vi "ASD PowerPoint Main.vi"() -> ()   [LabVIEW 2021]
uses:
  Controls/Functions Tab.ctl
  Controls/Channel Configuration List.ctl
  Controls/Channel Configuration Cluster.ctl
  Controls/Channel Configuration Cluster High Current.ctl
  Controls/Gain Array.ctl
  Controls/WT1800 Measurements.ctl
  Controls/WT1800 Readings.ctl
  Controls/Gain Averages.ctl
  Controls/Consumer Control.ctl
  Controls/Error Module Command.ctl
  Controls/DSA Readings.ctl
  Controls/Datalog Bundle Control.ctl
  Controls/WT1800 Functions.ctl
  Controls/DSA Functions.ctl
  Controls/DSA Measurements.ctl
panel:
  in  "User Gains":T1 {"Gain 6" format="%.2f"; "Gain 5" format="%.2f"; "Gain 4" format="%.2f"; "Gain 3" format="%.2f"; "Gain 2" min=-10.0 max=50.0 step=0.01 format="%.2f"; "Gain 1" min=-10.0 max=50.0 step=0.01 format="%.2f"}
  in  "Stop":bool
  in  "Home":bool
  in  "Abort":bool
  in  "Tab Control":T2
  in  "Power Test M":bool
  in  "Wave File 4":path
  in  "Wave File 3":path
  in  "Supply Set":bool
  in  "Temp Criteria":dbl caption="Temp Convergence Criteria [deg C]" min=0.0 max=10.0 step=0.01 format="%.2f"
  in  "Check EQ":bool
  in  "Load Settings":bool
  in  "Wave File 1":path
  in  "Voltage Steps":dbl[](array[numeric])=[0.0, 0.25, 0.5, 1.0, 1.95, 3.0, 3.9, 5.5] caption="Voltage Steps [Vrms]" min=0.0 max=500.0 step=0.01 format="%.2f"
  in  "User Notes":string
  in  "Supply Amps":dbl=50.0 caption="Max Supply Amps [Idc]" min=5.0 max=50.0 format="%.2f"
  in  "Supply Volts":dbl=14.4 caption="Supply Volts [Vdc]" min=10.0 max=15.0 format="%.2f"
  in  "Save Settings":bool
  in  "Configure Channels":bool
  in  "Exit":bool
  in  "Settling Delay":dbl=10.0 min=0.0 max=86400.0 format="%<%H:%M:%S>t"
  in  "Power Test":bool
  in  "Wave File 2":path
  in  "Data File":path caption="Data File Path"
  in  "Crest Factor":bool
  in  "Next Button":bool
  in  "Range":bool
  in  "Channel List":T3={"Channel Configuration Cluster"={"Input"=enum."---", "Enable"=FALSE, "User Notes"="", "Voltage Range"=15.0, "Current Range"=2.5}, "Channel Configuration Cluster 2"={"Input"=enum."---", "Enable"=FALSE, "User Notes"="", "Voltage Range"=15.0, "Current Range"=2.5}, "Channel Configuration Cluster 3"={"Input"=enum."---", "Enable"=FALSE, "User Notes"="", "Voltage Range"=15.0, "Current Range"=2.5}, "Channel Configuration Cluster 4"={"Input"=enum."---", "Enable"=FALSE, "User Notes"="", "Voltage Range"=15.0, "Current Range"=2.5}, "Channel Configuration Cluster 5"={"Input"=enum."---", "Enable"=FALSE, "User Notes"="", "Voltage Range"=15.0, "Current Range"=2.5}, "Channel Configuration Cluster 6"={"Input"=enum."---", "Enable"=FALSE, "User Notes"="", "Voltage Range"=15.0, "Current Range"=2.5}, "Channel Configuration Cluster 7"={"Input"=enum."---", "Enable"=FALSE, "User Notes"="", "Voltage Range"=15.0, "Current Range"=2.5}, "Channel Configuration Cluster 8"={"Input"=enum."---", "Enable"=FALSE, "User Notes"="", "Voltage Range"=15.0, "Current Range"=2.5}, "Channel Configuration Cluster 9"={"Input"=enum."---", "Enable"=FALSE, "User Notes"="", "Voltage Range"=15.0, "Current Range"=2.5}, "Channel Configuration Cluster 10"={"Input"=enum."---", "Enable"=FALSE, "User Notes"="", "Voltage Range"=15.0, "Current Range"=25.0}, "Channel Configuration Cluster 11"={"Input"=enum."---", "Enable"=FALSE, "User Notes"="", "Voltage Range"=15.0, "Current Range"=25.0}, "Channel Configuration Cluster 12"={"Input"=enum."---", "Enable"=FALSE, "User Notes"="", "Voltage Range"=15.0, "Current Range"=25.0}, "Channel Configuration Cluster 13"={"Input"=enum."---", "Enable"=FALSE, "User Notes"="", "Voltage Range"=15.0, "Current Range"=25.0}, "Channel Configuration Cluster 14"={"Input"=enum."---", "Enable"=FALSE, "User Notes"="", "Voltage Range"=15.0, "Current Range"=25.0}, "Channel Configuration Cluster 15"={"Input"=enum."---", "Enable"=FALSE, "User Notes"="", "Voltage Range"=15.0, "Current Range"=25.0}, "Channel Configuration Cluster 16"={"Input"=enum."---", "Enable"=FALSE, "User Notes"="", "Voltage Range"=15.0, "Current Range"=25.0}, "Channel Configuration Cluster 17"={"Input"=enum."---", "Enable"=FALSE, "User Notes"="", "Voltage Range"=15.0, "Current Range"=25.0}} {"Channel Configuration Cluster 17"."Current Range" items=["1 <500m>"=0.5, "2 <1>"=1.0, "5 <2.5>"=2.5, "10 <5>"=5.0, "20 <10>"=10.0, "50 <25>"=25.0]; "Channel Configuration Cluster 17"."Voltage Range" items=["1.5 <0.75>"=0.75, "3 <1.5>"=1.5, "6 <3>"=3.0, "10 <5>"=5.0, "15 <7.5>"=7.5, "30 <15>"=15.0, "60 <30>"=30.0, "100 <50>"=50.0, "150 <75>"=75.0, "300 <150>"=150.0, "600 <300>"=300.0, "1000 <500>"=500.0]; "Channel Configuration Cluster 16"."Current Range" items=["1 <500m>"=0.5, "2 <1>"=1.0, "5 <2.5>"=2.5, "10 <5>"=5.0, "20 <10>"=10.0, "50 <25>"=25.0]; "Channel Configuration Cluster 16"."Voltage Range" items=["1.5 <0.75>"=0.75, "3 <1.5>"=1.5, "6 <3>"=3.0, "10 <5>"=5.0, "15 <7.5>"=7.5, "30 <15>"=15.0, "60 <30>"=30.0, "100 <50>"=50.0, "150 <75>"=75.0, "300 <150>"=150.0, "600 <300>"=300.0, "1000 <500>"=500.0]; "Channel Configuration Cluster 15"."Current Range" items=["1 <500m>"=0.5, "2 <1>"=1.0, "5 <2.5>"=2.5, "10 <5>"=5.0, "20 <10>"=10.0, "50 <25>"=25.0]; "Channel Configuration Cluster 15"."Voltage Range" items=["1.5 <0.75>"=0.75, "3 <1.5>"=1.5, "6 <3>"=3.0, "10 <5>"=5.0, "15 <7.5>"=7.5, "30 <15>"=15.0, "60 <30>"=30.0, "100 <50>"=50.0, "150 <75>"=75.0, "300 <150>"=150.0, "600 <300>"=300.0, "1000 <500>"=500.0]; "Channel Configuration Cluster 14"."Current Range" items=["1 <500m>"=0.5, "2 <1>"=1.0, "5 <2.5>"=2.5, "10 <5>"=5.0, "20 <10>"=10.0, "50 <25>"=25.0]; "Channel Configuration Cluster 14"."Voltage Range" items=["1.5 <0.75>"=0.75, "3 <1.5>"=1.5, "6 <3>"=3.0, "10 <5>"=5.0, "15 <7.5>"=7.5, "30 <15>"=15.0, "60 <30>"=30.0, "100 <50>"=50.0, "150 <75>"=75.0, "300 <150>"=150.0, "600 <300>"=300.0, "1000 <500>"=500.0]; "Channel Configuration Cluster 13"."Current Range" items=["1 <500m>"=0.5, "2 <1>"=1.0, "5 <2.5>"=2.5, "10 <5>"=5.0, "20 <10>"=10.0, "50 <25>"=25.0]; "Channel Configuration Cluster 13"."Voltage Range" items=["1.5 <0.75>"=0.75, "3 <1.5>"=1.5, "6 <3>"=3.0, "10 <5>"=5.0, "15 <7.5>"=7.5, "30 <15>"=15.0, "60 <30>"=30.0, "100 <50>"=50.0, "150 <75>"=75.0, "300 <150>"=150.0, "600 <300>"=300.0, "1000 <500>"=500.0]; "Channel Configuration Cluster 12"."Current Range" items=["1 <500m>"=0.5, "2 <1>"=1.0, "5 <2.5>"=2.5, "10 <5>"=5.0, "20 <10>"=10.0, "50 <25>"=25.0]; "Channel Configuration Cluster 12"."Voltage Range" items=["1.5 <0.75>"=0.75, "3 <1.5>"=1.5, "6 <3>"=3.0, "10 <5>"=5.0, "15 <7.5>"=7.5, "30 <15>"=15.0, "60 <30>"=30.0, "100 <50>"=50.0, "150 <75>"=75.0, "300 <150>"=150.0, "600 <300>"=300.0, "1000 <500>"=500.0]; "Channel Configuration Cluster 11"."Current Range" items=["1 <500m>"=0.5, "2 <1>"=1.0, "5 <2.5>"=2.5, "10 <5>"=5.0, "20 <10>"=10.0, "50 <25>"=25.0]; "Channel Configuration Cluster 11"."Voltage Range" items=["1.5 <0.75>"=0.75, "3 <1.5>"=1.5, "6 <3>"=3.0, "10 <5>"=5.0, "15 <7.5>"=7.5, "30 <15>"=15.0, "60 <30>"=30.0, "100 <50>"=50.0, "150 <75>"=75.0, "300 <150>"=150.0, "600 <300>"=300.0, "1000 <500>"=500.0]; "Channel Configuration Cluster 10"."Current Range" items=["1 <500m>"=0.5, "2 <1>"=1.0, "5 <2.5>"=2.5, "10 <5>"=5.0, "20 <10>"=10.0, "50 <25>"=25.0]; "Channel Configuration Cluster 10"."Voltage Range" items=["1.5 <0.75>"=0.75, "3 <1.5>"=1.5, "6 <3>"=3.0, "10 <5>"=5.0, "15 <7.5>"=7.5, "30 <15>"=15.0, "60 <30>"=30.0, "100 <50>"=50.0, "150 <75>"=75.0, "300 <150>"=150.0, "600 <300>"=300.0, "1000 <500>"=500.0]; "Channel Configuration Cluster 9"."Voltage Range" items=["1.5 <0.75>"=0.75, "3 <1.5>"=1.5, "6 <3>"=3.0, "10 <5>"=5.0, "15 <7.5>"=7.5, "30 <15>"=15.0, "60 <30>"=30.0, "100 <50>"=50.0, "150 <75>"=75.0, "300 <150>"=150.0, "600 <300>"=300.0, "1000 <500>"=500.0]; "Channel Configuration Cluster 9"."Current Range" items=["10m <5m>"=0.005, "20m <10m>"=0.01, "50m <25m>"=0.025, "100m <50m>"=0.05, "200m <100m>"=0.1, "500m <250m>"=0.25, "1 <500m>"=0.5, "2 <1>"=1.0, "5 <2.5>"=2.5]; "Channel Configuration Cluster 8"."Voltage Range" items=["1.5 <0.75>"=0.75, "3 <1.5>"=1.5, "6 <3>"=3.0, "10 <5>"=5.0, "15 <7.5>"=7.5, "30 <15>"=15.0, "60 <30>"=30.0, "100 <50>"=50.0, "150 <75>"=75.0, "300 <150>"=150.0, "600 <300>"=300.0, "1000 <500>"=500.0]; "Channel Configuration Cluster 8"."Current Range" items=["10m <5m>"=0.005, "20m <10m>"=0.01, "50m <25m>"=0.025, "100m <50m>"=0.05, "200m <100m>"=0.1, "500m <250m>"=0.25, "1 <500m>"=0.5, "2 <1>"=1.0, "5 <2.5>"=2.5]; "Channel Configuration Cluster 7"."Voltage Range" items=["1.5 <0.75>"=0.75, "3 <1.5>"=1.5, "6 <3>"=3.0, "10 <5>"=5.0, "15 <7.5>"=7.5, "30 <15>"=15.0, "60 <30>"=30.0, "100 <50>"=50.0, "150 <75>"=75.0, "300 <150>"=150.0, "600 <300>"=300.0, "1000 <500>"=500.0]; "Channel Configuration Cluster 7"."Current Range" items=["10m <5m>"=0.005, "20m <10m>"=0.01, "50m <25m>"=0.025, "100m <50m>"=0.05, "200m <100m>"=0.1, "500m <250m>"=0.25, "1 <500m>"=0.5, "2 <1>"=1.0, "5 <2.5>"=2.5]; "Channel Configuration Cluster 6"."Voltage Range" items=["1.5 <0.75>"=0.75, "3 <1.5>"=1.5, "6 <3>"=3.0, "10 <5>"=5.0, "15 <7.5>"=7.5, "30 <15>"=15.0, "60 <30>"=30.0, "100 <50>"=50.0, "150 <75>"=75.0, "300 <150>"=150.0, "600 <300>"=300.0, "1000 <500>"=500.0]; "Channel Configuration Cluster 6"."Current Range" items=["10m <5m>"=0.005, "20m <10m>"=0.01, "50m <25m>"=0.025, "100m <50m>"=0.05, "200m <100m>"=0.1, "500m <250m>"=0.25, "1 <500m>"=0.5, "2 <1>"=1.0, "5 <2.5>"=2.5]; "Channel Configuration Cluster 5"."Voltage Range" items=["1.5 <0.75>"=0.75, "3 <1.5>"=1.5, "6 <3>"=3.0, "10 <5>"=5.0, "15 <7.5>"=7.5, "30 <15>"=15.0, "60 <30>"=30.0, "100 <50>"=50.0, "150 <75>"=75.0, "300 <150>"=150.0, "600 <300>"=300.0, "1000 <500>"=500.0]; "Channel Configuration Cluster 5"."Current Range" items=["10m <5m>"=0.005, "20m <10m>"=0.01, "50m <25m>"=0.025, "100m <50m>"=0.05, "200m <100m>"=0.1, "500m <250m>"=0.25, "1 <500m>"=0.5, "2 <1>"=1.0, "5 <2.5>"=2.5]; "Channel Configuration Cluster 4"."Voltage Range" items=["1.5 <0.75>"=0.75, "3 <1.5>"=1.5, "6 <3>"=3.0, "10 <5>"=5.0, "15 <7.5>"=7.5, "30 <15>"=15.0, "60 <30>"=30.0, "100 <50>"=50.0, "150 <75>"=75.0, "300 <150>"=150.0, "600 <300>"=300.0, "1000 <500>"=500.0]; "Channel Configuration Cluster 4"."Current Range" items=["10m <5m>"=0.005, "20m <10m>"=0.01, "50m <25m>"=0.025, "100m <50m>"=0.05, "200m <100m>"=0.1, "500m <250m>"=0.25, "1 <500m>"=0.5, "2 <1>"=1.0, "5 <2.5>"=2.5]; "Channel Configuration Cluster 3"."Voltage Range" items=["1.5 <0.75>"=0.75, "3 <1.5>"=1.5, "6 <3>"=3.0, "10 <5>"=5.0, "15 <7.5>"=7.5, "30 <15>"=15.0, "60 <30>"=30.0, "100 <50>"=50.0, "150 <75>"=75.0, "300 <150>"=150.0, "600 <300>"=300.0, "1000 <500>"=500.0]; "Channel Configuration Cluster 3"."Current Range" items=["10m <5m>"=0.005, "20m <10m>"=0.01, "50m <25m>"=0.025, "100m <50m>"=0.05, "200m <100m>"=0.1, "500m <250m>"=0.25, "1 <500m>"=0.5, "2 <1>"=1.0, "5 <2.5>"=2.5]; "Channel Configuration Cluster 2"."Voltage Range" items=["1.5 <0.75>"=0.75, "3 <1.5>"=1.5, "6 <3>"=3.0, "10 <5>"=5.0, "15 <7.5>"=7.5, "30 <15>"=15.0, "60 <30>"=30.0, "100 <50>"=50.0, "150 <75>"=75.0, "300 <150>"=150.0, "600 <300>"=300.0, "1000 <500>"=500.0]; "Channel Configuration Cluster 2"."Current Range" items=["10m <5m>"=0.005, "20m <10m>"=0.01, "50m <25m>"=0.025, "100m <50m>"=0.05, "200m <100m>"=0.1, "500m <250m>"=0.25, "1 <500m>"=0.5, "2 <1>"=1.0, "5 <2.5>"=2.5]; "Channel Configuration Cluster"."Voltage Range" items=["1.5 <0.75>"=0.75, "3 <1.5>"=1.5, "6 <3>"=3.0, "10 <5>"=5.0, "15 <7.5>"=7.5, "30 <15>"=15.0, "60 <30>"=30.0, "100 <50>"=50.0, "150 <75>"=75.0, "300 <150>"=150.0, "600 <300>"=300.0, "1000 <500>"=500.0]; "Channel Configuration Cluster"."Current Range" items=["10m <5m>"=0.005, "20m <10m>"=0.01, "50m <25m>"=0.025, "100m <50m>"=0.05, "200m <100m>"=0.1, "500m <250m>"=0.25, "1 <500m>"=0.5, "2 <1>"=1.0, "5 <2.5>"=2.5]}
  out "Gain Array":T6 {"Gain 17" format="%.2f"; "Gain 16" format="%.2f"; "Gain 15" format="%.2f"; "Gain 14" format="%.2f"; "Gain 13" format="%.2f"; "Gain 12" format="%.2f"; "Gain 11" format="%.2f"; "Gain 10" format="%.2f"; "Gain 9" format="%.2f"; "Gain 8" format="%.2f"; "Gain 7" format="%.2f"; "Gain 6" format="%.2f"; "Gain 5" format="%.2f"; "Gain 4" format="%.2f"; "Gain 3" format="%.2f"; "Gain 2" format="%.2f"; "Gain 1" format="%.2f"}
  out "Gain Averages":T1 {"Gain 6" format="%.2f"; "Gain 5" format="%.2f"; "Gain 4" format="%.2f"; "Gain 3" format="%.2f"; "Gain 2" format="%.2f"; "Gain 1" format="%.2f"}
  in  "Run Configuration":bool
  in  "Config Voltage":dbl=1.0 caption="Input Level\n[Vrms]" min=0.001 max=5.0 format="%.2f"
  out "Test Countdown 2":dbl caption="Test Count" min=0.0 max=86400.0 format="%<%H:%M:%S>t"
  in  "Manual Warning":bool=TRUE
  out "Temp":T7 caption="Themocouple Temperatures   °C" {"32" format="%.2f"; "31" format="%.2f"; "30" format="%.2f"; "29" format="%.2f"; "28" format="%.2f"; "27" format="%.2f"; "26" format="%.2f"; "25" format="%.2f"; "24" format="%.2f"; "23" format="%.2f"; "22" format="%.2f"; "21" format="%.2f"; "20" format="%.2f"; "19" format="%.2f"; "18" format="%.2f"; "17" format="%.2f"; "16" format="%.2f"; "15" format="%.2f"; "14" format="%.2f"; "13" format="%.2f"; "12" format="%.2f"; "11" format="%.2f"; "10" format="%.2f"; "9" format="%.2f"; "8" format="%.2f"; "7" format="%.2f"; "6" format="%.2f"; "5" format="%.2f"; "4" format="%.2f"; "3" format="%.2f"; "2" format="%.2f"; "1" format="%.2f"}
  out "Total":i32
  out "Current":i32
  out "Heat":dbl caption="Power Loss" min=1.0 step=1.0 format="%#.1f"
  out "Power Plot":i32=1 caption="Ch" min=1 step=1
  in  "P Scale":bool
  out "Test Countdown":dbl caption="Test Count" min=0.0 max=86400.0 format="%<%H:%M:%S>t"
  out "V Step":dbl caption="Voltage Step\n[Vrms]" format="%.2f"
  out "Delay Countdown":dbl caption="Delay Count" min=0.0 max=86400.0 format="%<%H:%M:%S>t"
  out "WT1800":T8 {"Vrms" format="%.3f"; "Irms" format="%.3f"; "Power" format="%.3f"; "Vpkpk" format="%.3f"; "Ipkpk" format="%.3f"}
  in  "Run Test":bool
  out "Power Graph":dbl[][](graph)
  in  "Auto Range":bool
  in  "Resolution":bool
  in  "Z Scale":bool
  in  "EQ Scale":bool
  out "Z Plot":i32=1 caption="Ch" min=1 step=1
  out "EQ Plot":i32=1 caption="Ch" min=1 step=1
  in  "Run EQ Check":bool
  in  "Abort 3":bool
  out "Frequency":dbl caption="Frequency [Hz]" format="%.2f"
  out "EQ Graph":cluster{dbl[], "Gain Array":dbl[]}[](graph)
  out "Z Graph":cluster{dbl[], "Gain Array":dbl[]}[](graph)
  # "OR"
  # "Gain1 [dB]"
  # "Gain2 [dB]"
  # "Gain3 [dB]"
  # "Gain4 [dB]"
  # "Gain [dB]"
  # "Save Data"
  # "Input"
  # "User Notes"
  # "1"
  # "2"
  # "3"
  # "4"
  # "5"
  # "6"
  # "7"
  # "8"
  # "9"
  # "10"
  # "11"
  # "12"
  # "13"
  # "14"
  # "15"
  # "16"
  # "17"
  # "User Gains [dB]"
  # "of"
  # "Supply Power    & Loss    [W]"
  # "Vrms"
  # "Irms"
  # "Watts"
  # "Vpp"
  # "Ipp"
  # "Output Power / Channel [W]"
  # "1"
  # "2"
  # "3"
  # "4"
  # "5"
  # "6"
  # "7"
  # "8"
  # "9"
  # "10"
  # "11"
  # "12"
  # "13"
  # "14"
  # "15"
  # "16"
  # "17"
  # "18"
  # "User Gains [dB]"
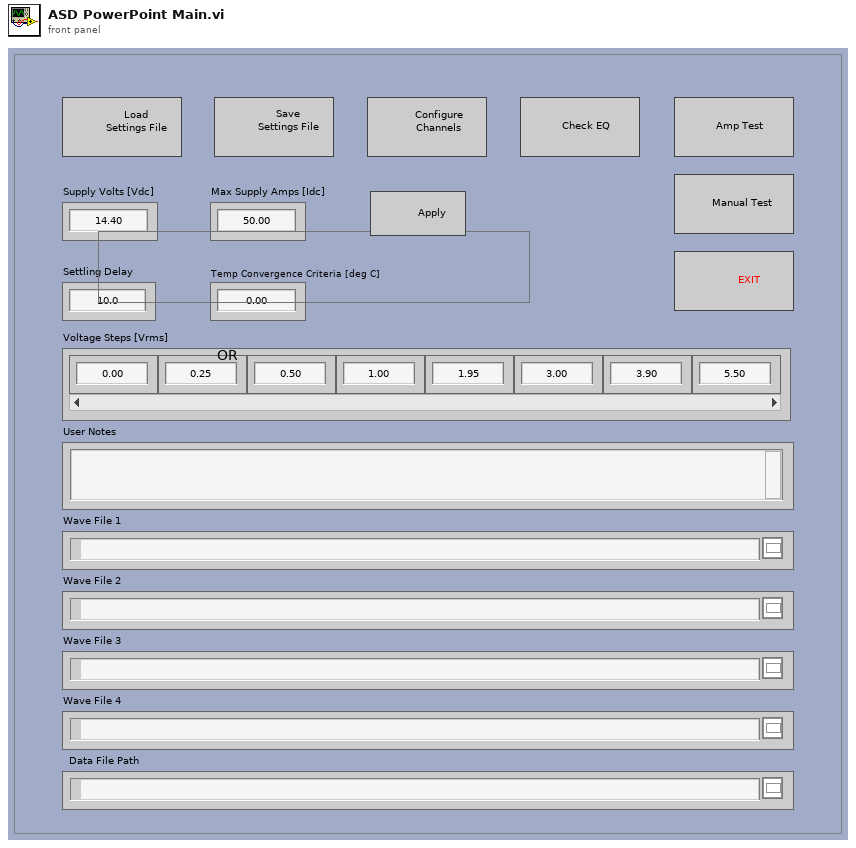
[diagram p1: front panel]
types:
  T1 = typedef "Gain Averages.ctl" = cluster{"Gain 1":dbl, "Gain 2":dbl, "Gain 3":dbl, "Gain 4":dbl, "Gain 5":dbl, "Gain 6":dbl}
  T2 = typedef "Functions Tab.ctl" = enum32{"Home", "Channel Configuration", "Power Test", "EQ Check"}
  T3 = typedef "Channel Configuration List.ctl" = cluster{"Channel Configuration Cluster":T4, "Channel Configuration Cluster 2":T4, "Channel Configuration Cluster 3":T4, "Channel Configuration Cluster 4":T4, "Channel Configuration Cluster 5":T4, "Channel Configuration Cluster 6":T4, "Channel Configuration Cluster 7":T4, "Channel Configuration Cluster 8":T4, "Channel Configuration Cluster 9":T4, "Channel Configuration Cluster 10":T5, "Channel Configuration Cluster 11":T5, "Channel Configuration Cluster 12":T5, "Channel Configuration Cluster 13":T5, "Channel Configuration Cluster 14":T5, "Channel Configuration Cluster 15":T5, "Channel Configuration Cluster 16":T5, "Channel Configuration Cluster 17":T5}
  T4 = typedef "Channel Configuration Cluster.ctl" = cluster{"Input":enum16{"---", "1", "1 AVG", "2", "2 AVG", "3", "3 AVG", "4", "4 AVG"}, "Enable":bool, "User Notes":string, "Voltage Range":dbl, "Current Range":dbl}
  T5 = typedef "Channel Configuration Cluster High Current.ctl" = cluster{"Input":enum16{"---", "1", "1 AVG", "2", "2 AVG", "3", "3 AVG", "4", "4 AVG"}, "Enable":bool, "User Notes":string, "Voltage Range":dbl, "Current Range":dbl}
  T6 = typedef "Gain Array.ctl" = cluster{"Gain 1":dbl, "Gain 2":dbl, "Gain 3":dbl, "Gain 4":dbl, "Gain 5":dbl, "Gain 6":dbl, "Gain 7":dbl, "Gain 8":dbl, "Gain 9":dbl, "Gain 10":dbl, "Gain 11":dbl, "Gain 12":dbl, "Gain 13":dbl, "Gain 14":dbl, "Gain 15":dbl, "Gain 16":dbl, "Gain 17":dbl}
  T7 = cluster{"1":sgl, "2":sgl, "3":sgl, "4":sgl, "5":sgl, "6":sgl, "7":sgl, "8":sgl, "9":sgl, "10":sgl, "11":sgl, "12":sgl, "13":sgl, "14":sgl, "15":sgl, "16":sgl, "17":sgl, "18":sgl, "19":sgl, "20":sgl, "21":sgl, "22":sgl, "23":sgl, "24":sgl, "25":sgl, "26":sgl, "27":sgl, "28":sgl, "29":sgl, "30":sgl, "31":sgl, "32":sgl}
  T8 = typedef "WT1800 Measurements.ctl" = T9[]
  T9 = typedef "WT1800 Readings.ctl" = cluster{"Vrms":sgl, "Irms":sgl, "Power":sgl, "Vpkpk":sgl, "Ipkpk":sgl}
  T10 = typedef "Error Module Command.ctl" = enum16{"Initialize", "Handle Errors", "Report Errors"}
  T11 = typedef "Consumer Control.ctl" = cluster{"Command":enum16{"Initialize", "Home", "Configure Channels", "Fixed Range", "Set DC Supply", "Save Settings", "Load Settings", "Power Test", "Power Test M", "Run Configuration", "Run Test", "Abort", "Run EQ", "Check EQ", "Help", "Exit"}, "Data":variant}
  T12 = enum8{"Enabled", "Disabled", "Disabled and Grayed Out"}
  T13 = typedef "DSA Readings.ctl" = cluster{"Vrms":sgl, "Vdc":sgl, "Vpk+":sgl, "Vpk-":sgl, "Vpkpk":sgl}
  T14 = cluster{"1":dbl, "2":dbl, "3":dbl, "4":dbl, "5":dbl, "6":dbl, "7":dbl, "8":dbl, "9":dbl, "10":dbl, "11":dbl, "12":dbl, "13":dbl, "14":dbl, "15":dbl, "16":dbl, "17":dbl, "18":dbl, "19":dbl, "20":dbl, "21":dbl, "22":dbl, "23":dbl, "24":dbl, "25":dbl, "26":dbl, "27":dbl, "28":dbl, "29":dbl, "30":dbl, "31":dbl, "32":dbl}
  T15 = typedef "Datalog Bundle Control.ctl" = cluster{"Heat":dbl, "WT1800 Functions":T16, "WT1800 Averages":T8, "WT1800 Measurements":T9[][], "DSA Functions":T17, "DSA Averages":T18, "DSA Measurements":T13[][], "Initial Time Stamp":timestamp, "Final Time Stamp":timestamp, "Temperature Data":sgl[][]}
  T16 = typedef "WT1800 Functions.ctl" = cluster{"Channel":string, "Vrms":string, "Power":string, "Vpkpk":string, "Ipkpk":string, "Vpkpk":string}[]
  T17 = typedef "DSA Functions.ctl" = cluster{"Channel":string, "Vrms":string, "Vdc":string, "Vpk+":string, "Vpk-":string, "Vpkpk":string}[]
  T18 = typedef "DSA Measurements.ctl" = T13[]
  T19 = cluster{"Supply Volts":dbl, "Supply Amps":dbl, "Settling Delay":dbl, "Temp Criteria":dbl, "Voltage Steps":dbl[], "User Notes":string, "Data File":path, "Config Voltage":dbl, "Channel List":T3, "User Gains":T1, "Gain Averages":T1, "Gain Array":T6, "Wave File 1":path, "Wave File 2":path, "Wave File 3":path, "Wave File 4":path, "Range":bool, "Crest Factor":bool}
  T20 = enum16{"Initialize", "Home", "Configure Channels", "Fixed Range", "Set DC Supply", "Save Settings", "Load Settings", "Power Test", "Power Test M", "Run Configuration", "Run Test", "Abort", "Run EQ", "Check EQ", "Help", "Exit"}
  T21 = typedef "Settings Control.ctl" = cluster{"Supply Voltage [Vdc]":sgl, "Max Supply Current [Idc]":sgl, "Settling Delay":dbl, "Temp Criteria":sgl, "Voltage Steps [Vrms]":sgl[], "User Notes":string, "Config Wave File Path":path, "Config Voltage [Vrms]":sgl, "Channel Configuration List":T3, "User Gains":T1, "Gains":T1, "Gain Array":T6, "Wave File Path 1":path, "Wave File Path 2":path, "Wave File Path 3":path, "Wave File Path 4":path, "Range":bool, "CF":bool}
  T22 = typedef "Wave Generator Control.ctl" = cluster{"Signal Amplitude [Vrms]":dbl, "Signal Type":u16, "Frequency Range [Hz]":cluster{"start":dbl, "stop":dbl}, "Waveform Duration [Seconds]":dbl}
  T23 = cluster{"AO Task ID In":refnum<k21>[], "task out":refnum<k21>}
  T24 = cluster{"Temperature Data[0]":sgl, "Temperature Data[1]":sgl, "Temperature Data[2]":sgl, "Temperature Data[3]":sgl, "Temperature Data[4]":sgl, "Temperature Data[5]":sgl, "Temperature Data[6]":sgl, "Temperature Data[7]":sgl, "Temperature Data[8]":sgl, "Temperature Data[9]":sgl, "Temperature Data[10]":sgl, "Temperature Data[11]":sgl, "Temperature Data[12]":sgl, "Temperature Data[13]":sgl, "Temperature Data[14]":sgl, "Temperature Data[15]":sgl, "Temperature Data[16]":sgl, "Temperature Data[17]":sgl, "Temperature Data[18]":sgl, "Temperature Data[19]":sgl, "Temperature Data[20]":sgl, "Temperature Data[21]":sgl, "Temperature Data[22]":sgl, "Temperature Data[23]":sgl, "Temperature Data[24]":sgl, "Temperature Data[25]":sgl, "Temperature Data[26]":sgl, "Temperature Data[27]":sgl, "Temperature Data[28]":sgl, "Temperature Data[29]":sgl, "Temperature Data[30]":sgl, "Temperature Data[31]":sgl}
  T25 = typedef "imagedata.ctl" = cluster{"image type":i32, "image depth":i32, "image":u8[], "mask":u8[], "colors":u32[], "Rectangle":cluster{"left":i16, "top":i16, "right":i16, "bottom":i16}}
  T26 = enum16{"---", "1", "1 AVG", "2", "2 AVG", "3", "3 AVG", "4", "4 AVG"}
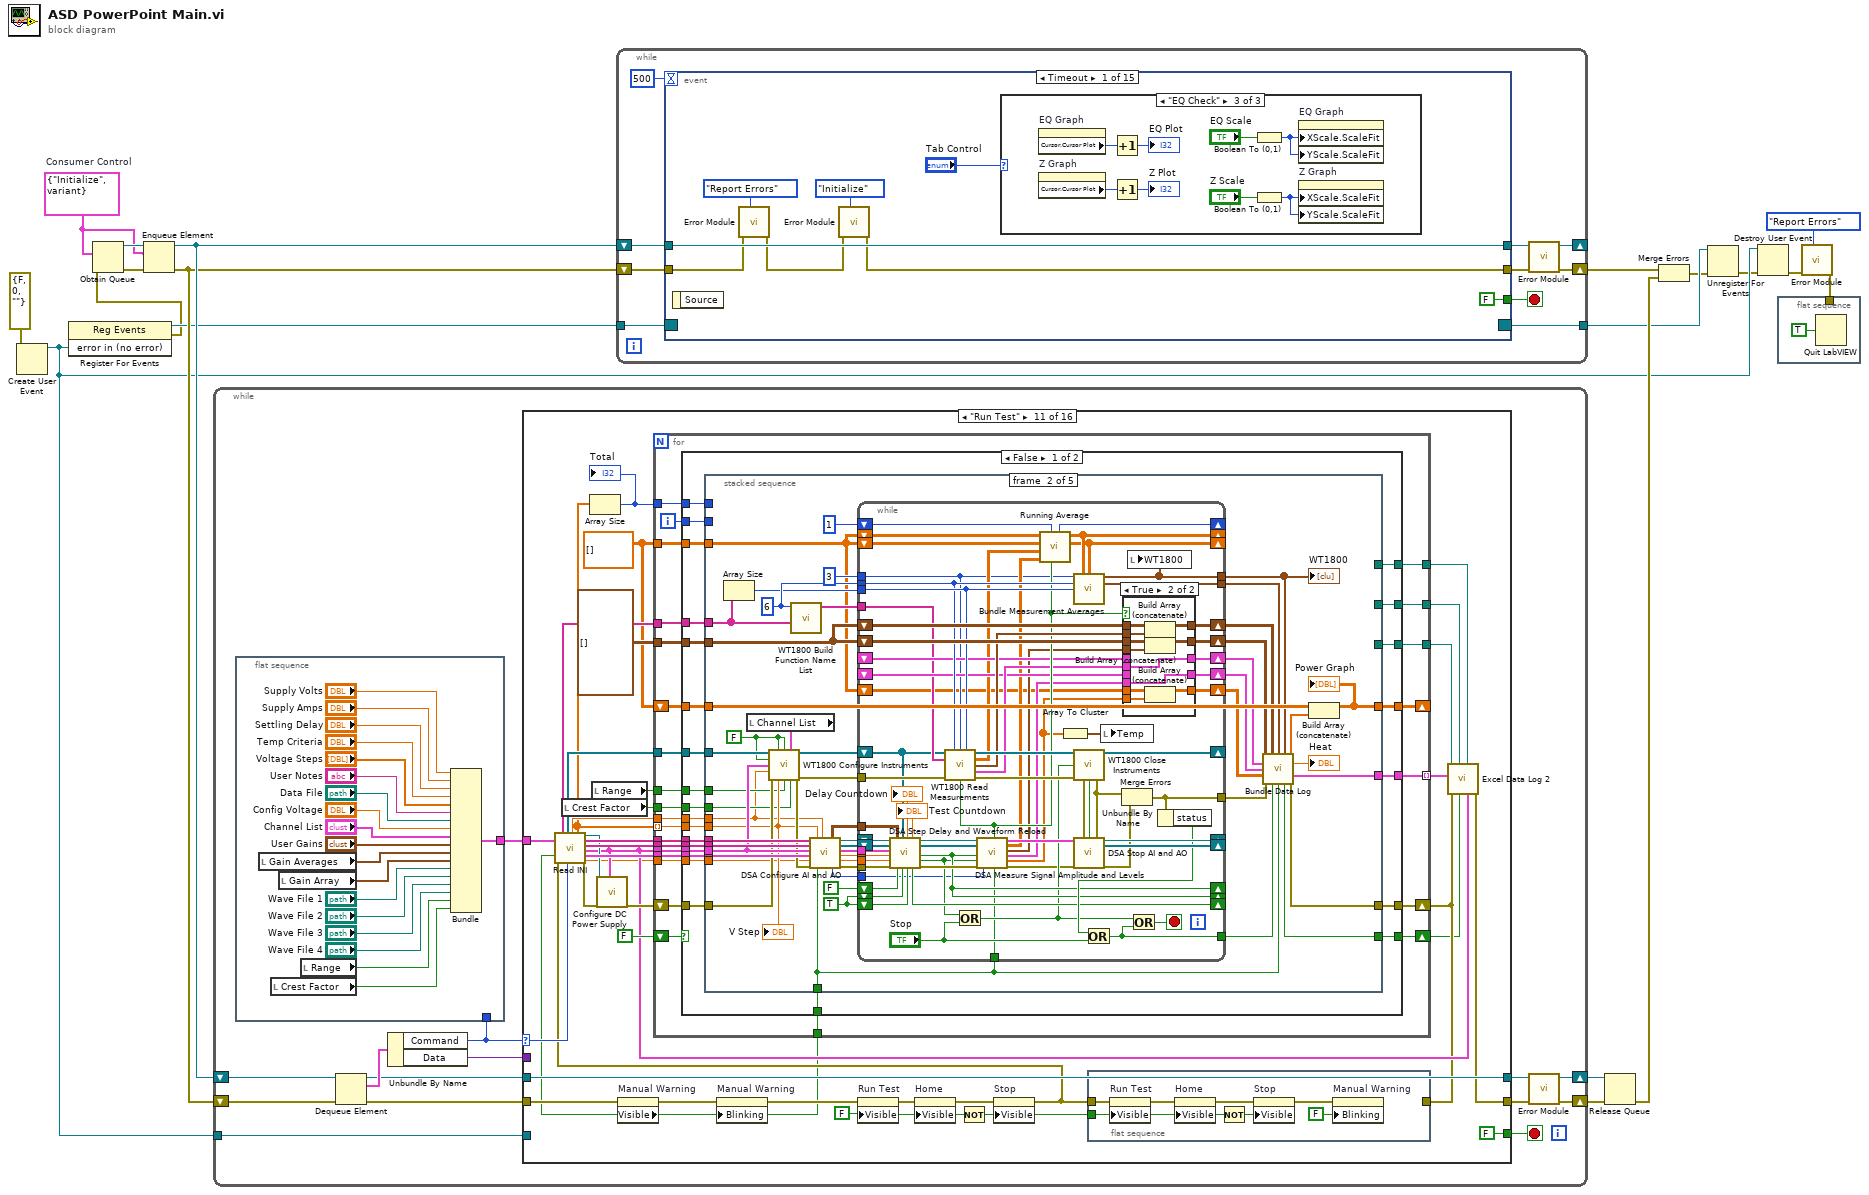
[diagram p0: block diagram]
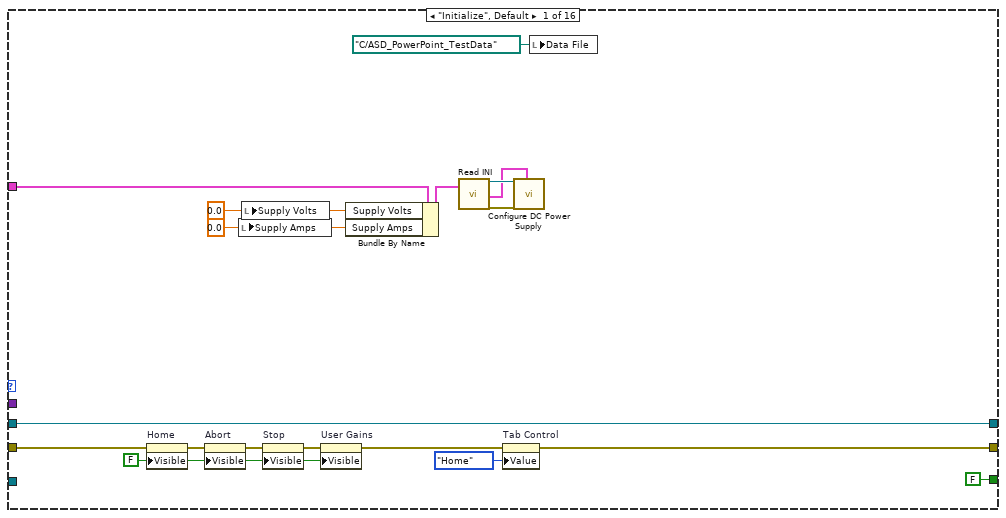
[diagram p2: hidden frame]
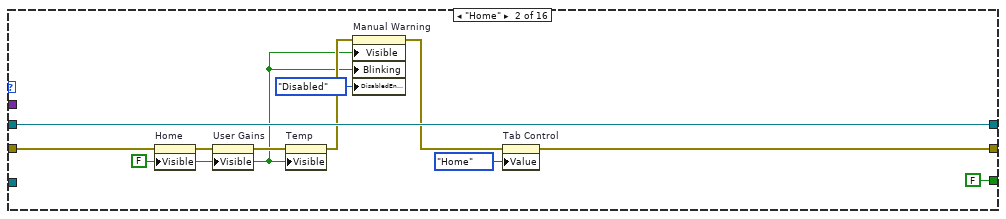
[diagram p3: hidden frame]
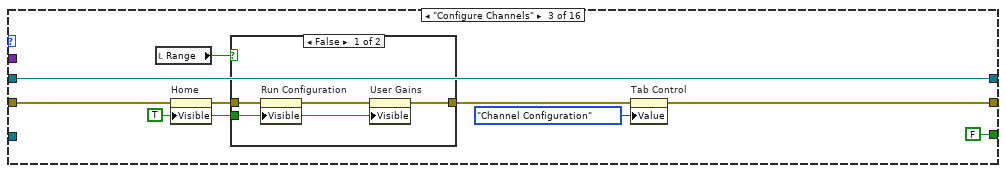
[diagram p4: hidden frame]
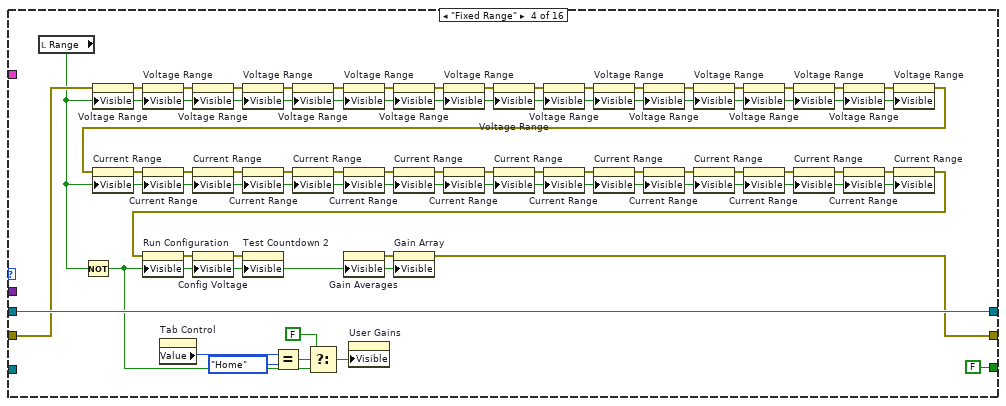
[diagram p6: hidden frame]
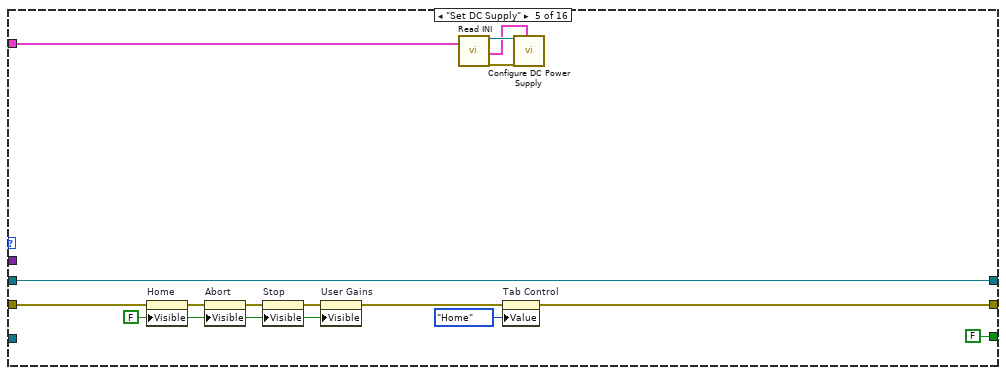
[diagram p7: hidden frame]
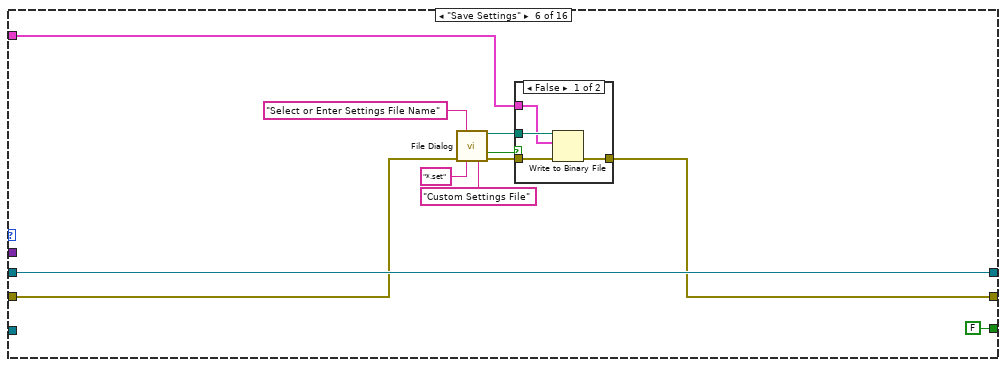
[diagram p8: hidden frame]
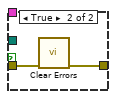
[diagram p9: hidden frame]
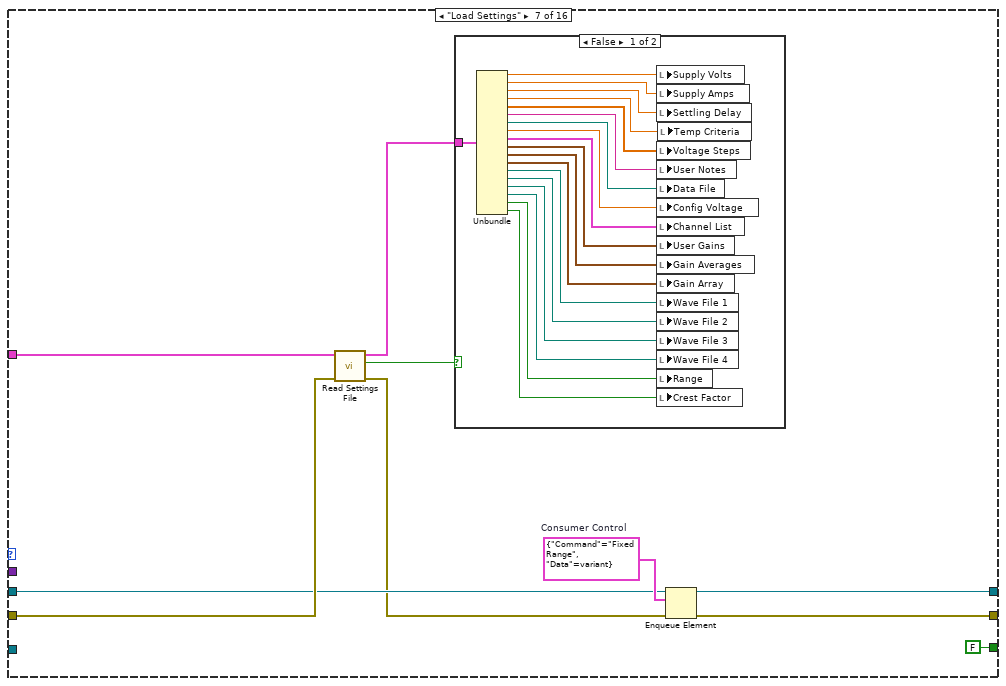
[diagram p10: hidden frame]
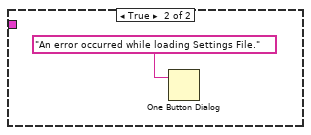
[diagram p11: hidden frame]
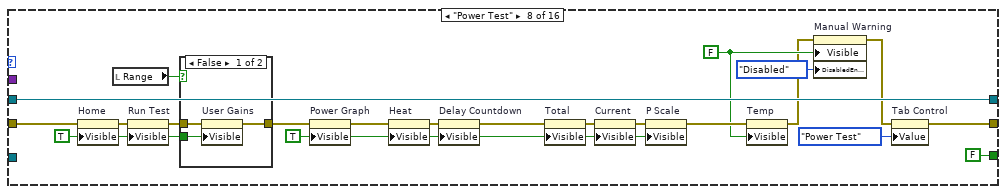
[diagram p12: hidden frame]
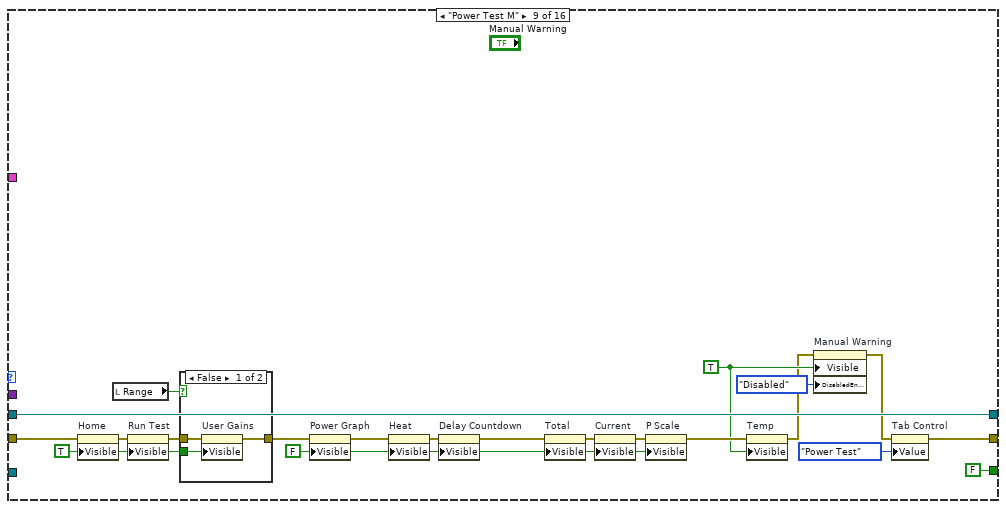
[diagram p14: hidden frame]
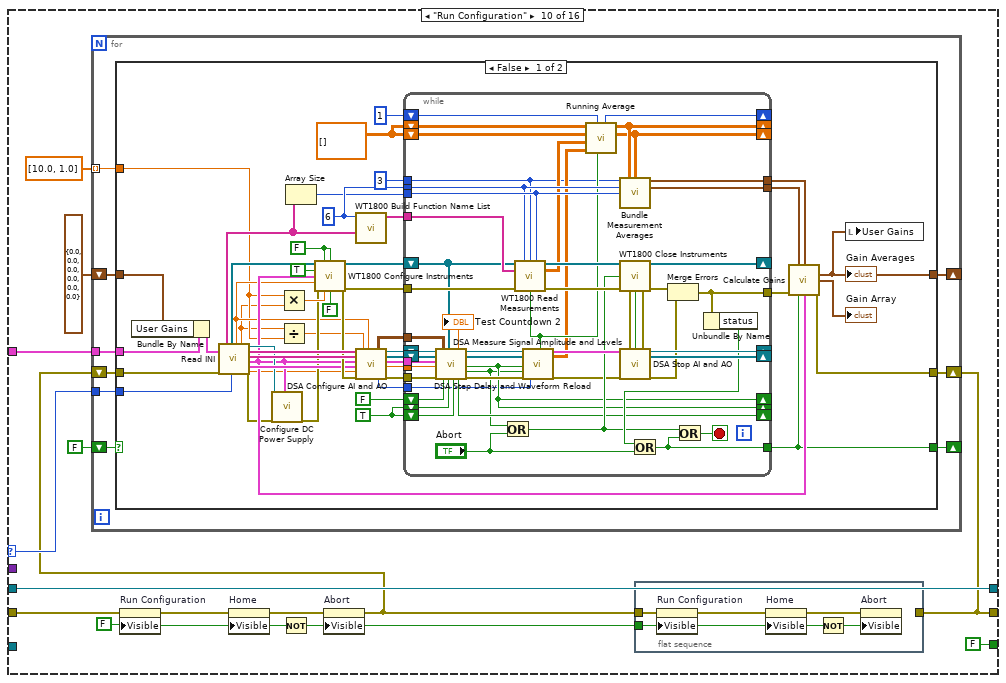
[diagram p16: hidden frame]
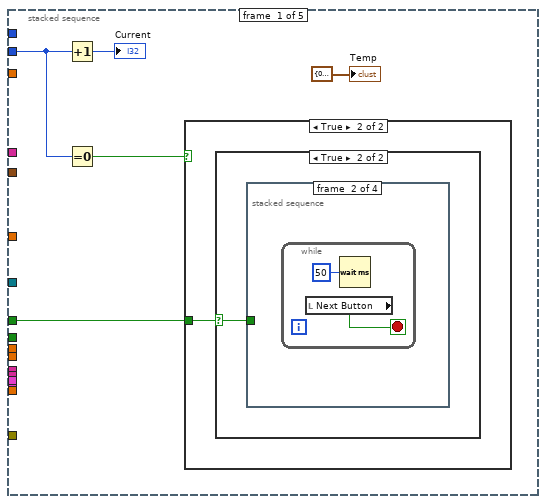
[diagram p18: hidden frame]
diagram:
  w2 = T11 {"Command"=enum."Initialize", "Data"=variant}  # Consumer Control
  n1 = Create User Event(user event datatype=errorcluster {"status"=FALSE, "code"=0, "source"=""} ("error in (no error)")) -> (user event=w7:refnum<user-event>)  [unwired: 1 in, 1 out]
  n2 = register-events(w7) -> (reference out=w10:refnum<event-registration>, error out=w8:errorcluster)  [unwired: 2 in]
  n3 = Obtain Queue(element data type=w2, error in (no error)=w8) -> (queue out=w19:refnum<queue>, error out=w16:errorcluster)  [unwired: 3 in, 1 out]
  n4 = Enqueue Element(queue=w19, element=w2, error in (no error)=w16) -> (queue out=w18:refnum<queue>, error out=w17:errorcluster)  [unwired: 1 in, 1 out]
  n5 = while {
    shift-right: [w26] -> w14
    shift-left: w18 -> [w32]
    shift-right: [w23] -> w13
    shift-left: w17 -> [w31]
    tunnel: w7 -> [w24]
    stop <- w28 stop-if-true
    n6 = flat-sequence {
      tunnel: [w51] -> w21
      tunnel: w20 -> [_]
      frame #0 {
        n7 = local read "Gain Averages"() -> (w42:T1)
        n8 = local read "Crest Factor"() -> (w34:bool)
        n9 = local read "Gain Array"() -> (w40:T6)
        n10 = local read "Range"() -> (w35:bool)
        n11 = Bundle("Supply Volts"="Supply Volts", "Supply Amps"="Supply Amps", "Settling Delay"="Settling Delay", "Temp Criteria"="Temp Criteria", "Voltage Steps"="Voltage Steps", "User Notes"="User Notes", "Data File"="Data File", "Config Voltage"="Config Voltage", "Channel List"="Channel List", "User Gains"="User Gains", "Gain Averages"=w42, "Gain Array"=w40, "Wave File 1"="Wave File 1", "Wave File 2"="Wave File 2", "Wave File 3"="Wave File 3", "Wave File 4"="Wave File 4", "Range"=w35, "Crest Factor"=w34) -> (w51:T19)  [unwired: 1 in]
      }
    }
    n12 = Dequeue Element(queue=w32, error in (no error)=w31) -> (queue out=w27:refnum<queue>, element=w30:T11, error out=w25:errorcluster)  [unwired: 1 in, 1 out]
    n13 = Unbundle By Name(w30) -> ("Command"=w20:T20, "Data"=w29:variant)
    n14 = case shown="\"Run Test\"" w20 {
      selector: w20 -> [_ _ _ _ _ _ _ _ _ w260 w405 _ w709 _ _ _]
      tunnel: w29 -> [_ _ _ _ _ _ _ _ _ _ _ _ _ _ _ _]
      tunnel: [FALSE FALSE FALSE FALSE FALSE FALSE FALSE FALSE FALSE FALSE FALSE FALSE FALSE FALSE FALSE TRUE] -> w28
      tunnel: w27 -> [w69 w80 w89 w142 w156 w167 w178 w224 w249 w267 w418 w685 w721 w889 w892 w902]
      tunnel: [w69 w80 w89 w142 w156 w167 w177 w224 w249 w267 w418 w685 w721 w889 w892 w902] -> w26
      tunnel: [w67 w78 w88 w101 w154 w157 w174 w223 w248 w256 w387 w684 w687 w888 w891 w901] -> w22
      tunnel: w25 -> [w65 w76 w86 w114 w152 w164 w182 w221 w246 w263 w383 w684 w716 w886 w891 w901]
      tunnel: w24 -> [_ _ _ _ _ _ _ _ _ _ _ _ _ _ _ _]
      tunnel: w21 -> [w56 _ _ _ w143 w158 w176 _ _ w259 w404 _ w713 _ _ w894]
      frame "Initialize", Default {
        w52 = 0.0 ("Supply Amps")
        w53 = 0.0 ("Supply Volts")
        w61 = FALSE ("Visible")
        n15 = property on="Home" class="Bool"(error in=w65, "Visible"=w61) -> (error out=w63:errorcluster)  [unwired: 1 in, 1 out]
        n16 = property on="Abort" class="Bool"(error in=w63, "Visible"=w61) -> (error out=w64:errorcluster)  [unwired: 1 in, 1 out]
        n17 = local write "Supply Amps"(w52) -> ()
        n18 = local write "Supply Volts"(w53) -> ()
        n19 = property on="Stop" class="Bool"(error in=w64, "Visible"=w61) -> (error out=w62:errorcluster)  [unwired: 1 in, 1 out]
        n20 = property on="User Gains" class="Clust (strict)"(error in=w62, "Visible"=w61) -> (error out=w60:errorcluster)  [unwired: 1 in, 1 out]
        n21 = Bundle By Name(cluster=w56, "Supply Volts"=w53, "Supply Amps"=w52) -> (w55:T19)
        n22 = call "Read INI.vi"("Settings Cluster In"=w55) -> ("DC Power Supply"=w58:refnum<visa-resource-name>, "Settings Cluster Out"=w57:T21, "Error Out"=w59:errorcluster)  [unwired: 6 in, 10 out]
        n23 = property on="Tab Control" class="TabCtl (strict)"(error in=w60, "Value"=Functions_Tab."Home" ("Tab Control")) -> (error out=w67:errorcluster)  [unwired: 1 in, 1 out]
        n24 = call "Configure DC Power Supply.vi"("DC Power Supply In"=w58, "Error In"=w59, "Settings Cluster"=w57) -> ()  [unwired: 15 in, 2 out]
        n25 = local write "Data File"(path "C:/ASD_PowerPoint_TestData" ("Data File")) -> ()
      }
      frame "Home" {
        w70 = FALSE ("Visible")
        n26 = property on="Home" class="Bool"(error in=w76, "Visible"=w70) -> (error out=w75:errorcluster)  [unwired: 1 in, 1 out]
        n27 = property on="User Gains" class="Clust (strict)"(error in=w75, "Visible"=w70) -> (error out=w72:errorcluster)  [unwired: 1 in, 1 out]
        n28 = property on="Temp" class="Clust (strict)"(error in=w72, "Visible"=w70) -> (error out=w74:errorcluster)  [unwired: 1 in, 1 out]
        n29 = property on="Manual Warning" class="Bool"(error in=w74, "Visible"=w70, "Blinking"=w70, "DisabledEnum"=T12."Disabled" ("Disabled")) -> (error out=w71:errorcluster)  [unwired: 1 in, 1 out]
        n30 = property on="Tab Control" class="TabCtl (strict)"(error in=w71, "Value"=Functions_Tab."Home" ("Tab Control")) -> (error out=w78:errorcluster)  [unwired: 1 in, 1 out]
      }
      frame "Configure Channels" {
        w82 = TRUE ("Visible")
        n31 = local read "Range"() -> (w81:bool)
        n32 = property on="Home" class="Bool"(error in=w86, "Visible"=w82) -> (error out=w84:errorcluster)  [unwired: 1 in, 1 out]
        n33 = case shown="False" w81 {
          tunnel: w84 -> [w93 w94]
          tunnel: [w91 w94] -> w83
          tunnel: w82 -> [w90 _]
          frame False {
            n34 = property on="Run Configuration" class="Bool"(error in=w93, "Visible"=w90) -> (error out=w92:errorcluster)  [unwired: 1 in, 1 out]
            n35 = property on="User Gains" class="Clust (strict)"(error in=w92, "Visible"=w90) -> (error out=w91:errorcluster)  [unwired: 1 in, 1 out]
          }
          frame True {
          }
        }
        n36 = property on="Tab Control" class="TabCtl (strict)"(error in=w83, "Value"=Functions_Tab."Channel Configuration" ("Tab Control")) -> (error out=w88:errorcluster)  [unwired: 1 in, 1 out]
      }
      frame "Fixed Range" {
        n37 = local read "Range"() -> (w106:bool)
        n38 = Not(x=w106) -> (.not. x?=w96:bool)
        n39 = property on="Voltage Range" class="Ring (strict)"(error in=w114, "Visible"=w106) -> (error out=w140:errorcluster)  [unwired: 1 in, 1 out]
        n40 = property on="Voltage Range" class="Ring (strict)"(error in=w140, "Visible"=w106) -> (error out=w139:errorcluster)  [unwired: 1 in, 1 out]
        n41 = property on="Tab Control" class="TabCtl (strict)"() -> ("Value"=w98:T2)  [unwired: 2 in, 2 out]
        n42 = property on="Voltage Range" class="Ring (strict)"(error in=w139, "Visible"=w106) -> (error out=w138:errorcluster)  [unwired: 1 in, 1 out]
        n43 = property on="Voltage Range" class="Ring (strict)"(error in=w138, "Visible"=w106) -> (error out=w137:errorcluster)  [unwired: 1 in, 1 out]
        n44 = Equal?(x=w98, y=Functions_Tab."Home" ("Tab Control")) -> (x = y?=w97:bool)
        n45 = property on="Voltage Range" class="Ring (strict)"(error in=w137, "Visible"=w106) -> (error out=w136:errorcluster)  [unwired: 1 in, 1 out]
        n46 = Select(t=FALSE, s=w97, f=w96) -> (s? t:f=w100:bool)
        n47 = property on="Voltage Range" class="Ring (strict)"(error in=w136, "Visible"=w106) -> (error out=w135:errorcluster)  [unwired: 1 in, 1 out]
        n48 = property on="Gain Averages" class="Clust (strict)"("Visible"=w96) -> (error out=w102:errorcluster)  [unwired: 2 in, 1 out]
        n49 = property on="User Gains" class="Clust (strict)"("Visible"=w100) -> ()  [unwired: 2 in, 2 out]
        n50 = property on="Voltage Range" class="Ring (strict)"(error in=w135, "Visible"=w106) -> (error out=w126:errorcluster)  [unwired: 1 in, 1 out]
        n51 = property on="Gain Array" class="Clust (strict)"(error in=w102, "Visible"=w96) -> (error out=w101:errorcluster)  [unwired: 1 in, 1 out]
        n52 = property on="Voltage Range" class="Ring (strict)"(error in=w126, "Visible"=w106) -> (error out=w125:errorcluster)  [unwired: 1 in, 1 out]
        n53 = property on="Voltage Range" class="Ring (strict)"(error in=w125, "Visible"=w106) -> (error out=w134:errorcluster)  [unwired: 1 in, 1 out]
        n54 = property on="Voltage Range" class="Ring (strict)"(error in=w134, "Visible"=w106) -> (error out=w133:errorcluster)  [unwired: 1 in, 1 out]
        n55 = property on="Voltage Range" class="Ring (strict)"(error in=w133, "Visible"=w106) -> (error out=w132:errorcluster)  [unwired: 1 in, 1 out]
        n56 = property on="Voltage Range" class="Ring (strict)"(error in=w132, "Visible"=w106) -> (error out=w131:errorcluster)  [unwired: 1 in, 1 out]
        n57 = property on="Voltage Range" class="Ring (strict)"(error in=w131, "Visible"=w106) -> (error out=w130:errorcluster)  [unwired: 1 in, 1 out]
        n58 = property on="Voltage Range" class="Ring (strict)"(error in=w130, "Visible"=w106) -> (error out=w129:errorcluster)  [unwired: 1 in, 1 out]
        n59 = property on="Voltage Range" class="Ring (strict)"(error in=w129, "Visible"=w106) -> (error out=w128:errorcluster)  [unwired: 1 in, 1 out]
        n60 = property on="Voltage Range" class="Ring (strict)"(error in=w128, "Visible"=w106) -> (error out=w127:errorcluster)  [unwired: 1 in, 1 out]
        n61 = property on="Voltage Range" class="Ring (strict)"(error in=w127, "Visible"=w106) -> (error out=w107:errorcluster)  [unwired: 1 in, 1 out]
        n62 = property on="Current Range" class="Ring (strict)"(error in=w107, "Visible"=w106) -> (error out=w124:errorcluster)  [unwired: 1 in, 1 out]
        n63 = property on="Current Range" class="Ring (strict)"(error in=w124, "Visible"=w106) -> (error out=w123:errorcluster)  [unwired: 1 in, 1 out]
        n64 = property on="Current Range" class="Ring (strict)"(error in=w123, "Visible"=w106) -> (error out=w122:errorcluster)  [unwired: 1 in, 1 out]
        n65 = property on="Current Range" class="Ring (strict)"(error in=w122, "Visible"=w106) -> (error out=w121:errorcluster)  [unwired: 1 in, 1 out]
        n66 = property on="Current Range" class="Ring (strict)"(error in=w121, "Visible"=w106) -> (error out=w120:errorcluster)  [unwired: 1 in, 1 out]
        n67 = property on="Current Range" class="Ring (strict)"(error in=w120, "Visible"=w106) -> (error out=w119:errorcluster)  [unwired: 1 in, 1 out]
        n68 = property on="Current Range" class="Ring (strict)"(error in=w119, "Visible"=w106) -> (error out=w118:errorcluster)  [unwired: 1 in, 1 out]
        n69 = property on="Current Range" class="Ring (strict)"(error in=w118, "Visible"=w106) -> (error out=w117:errorcluster)  [unwired: 1 in, 1 out]
        n70 = property on="Current Range" class="Ring (strict)"(error in=w117, "Visible"=w106) -> (error out=w116:errorcluster)  [unwired: 1 in, 1 out]
        n71 = property on="Current Range" class="Ring (strict)"(error in=w116, "Visible"=w106) -> (error out=w115:errorcluster)  [unwired: 1 in, 1 out]
        n72 = property on="Current Range" class="Ring (strict)"(error in=w115, "Visible"=w106) -> (error out=w113:errorcluster)  [unwired: 1 in, 1 out]
        n73 = property on="Current Range" class="Ring (strict)"(error in=w113, "Visible"=w106) -> (error out=w112:errorcluster)  [unwired: 1 in, 1 out]
        n74 = property on="Current Range" class="Ring (strict)"(error in=w112, "Visible"=w106) -> (error out=w111:errorcluster)  [unwired: 1 in, 1 out]
        n75 = property on="Current Range" class="Ring (strict)"(error in=w111, "Visible"=w106) -> (error out=w110:errorcluster)  [unwired: 1 in, 1 out]
        n76 = property on="Current Range" class="Ring (strict)"(error in=w110, "Visible"=w106) -> (error out=w109:errorcluster)  [unwired: 1 in, 1 out]
        n77 = property on="Current Range" class="Ring (strict)"(error in=w109, "Visible"=w106) -> (error out=w108:errorcluster)  [unwired: 1 in, 1 out]
        n78 = property on="Current Range" class="Ring (strict)"(error in=w108, "Visible"=w106) -> (error out=w105:errorcluster)  [unwired: 1 in, 1 out]
        n79 = property on="Run Configuration" class="Bool"(error in=w105, "Visible"=w96) -> (error out=w104:errorcluster)  [unwired: 1 in, 1 out]
        n80 = property on="Config Voltage" class="DigNum (strict)"(error in=w104, "Visible"=w96) -> (error out=w103:errorcluster)  [unwired: 1 in, 1 out]
        n81 = property on="Test Countdown 2" class="DigNum (strict)"(error in=w103, "Visible"=w96) -> ()  [unwired: 1 in, 2 out]
      }
      frame "Set DC Supply" {
        w148 = FALSE ("Visible")
        n82 = property on="Home" class="Bool"(error in=w152, "Visible"=w148) -> (error out=w150:errorcluster)  [unwired: 1 in, 1 out]
        n83 = property on="Abort" class="Bool"(error in=w150, "Visible"=w148) -> (error out=w151:errorcluster)  [unwired: 1 in, 1 out]
        n84 = property on="Stop" class="Bool"(error in=w151, "Visible"=w148) -> (error out=w149:errorcluster)  [unwired: 1 in, 1 out]
        n85 = property on="User Gains" class="Clust (strict)"(error in=w149, "Visible"=w148) -> (error out=w147:errorcluster)  [unwired: 1 in, 1 out]
        n86 = call "Read INI.vi"("Settings Cluster In"=w143) -> ("DC Power Supply"=w145:refnum<visa-resource-name>, "Settings Cluster Out"=w144:T21, "Error Out"=w146:errorcluster)  [unwired: 6 in, 10 out]
        n87 = property on="Tab Control" class="TabCtl (strict)"(error in=w147, "Value"=Functions_Tab."Home" ("Tab Control")) -> (error out=w154:errorcluster)  [unwired: 1 in, 1 out]
        n88 = call "Configure DC Power Supply.vi"("DC Power Supply In"=w145, "Error In"=w146, "Settings Cluster"=w144) -> ()  [unwired: 15 in, 2 out]
      }
      frame "Save Settings" {
        n89 = call "File Dialog"("prompt"="Select or Enter Settings File Name", "error in"=w164, "pattern (all files)"="*.set", "pattern label"="Custom Settings File") -> ("selected path"=w166:path, "cancelled"=w160:bool, "error out"=w165:errorcluster)  [unwired: 8 in, 1 out]
        n90 = case shown="False" w160 {
          tunnel: [w169 w172] -> w157
          tunnel: w166 -> [w171 _]
          tunnel: w165 -> [w170 w173]
          tunnel: w158 -> [w168 _]
          frame False {
            n91 = Write to Binary File(file (use dialog)=w171, data=w168, error in=w170) -> (error out=w169:errorcluster)  [unwired: 3 in, 2 out]
          }
          frame True {
            n92 = call <vilib>:"Clear Errors.vi"("error in (no error)"=w173) -> ("error out"=w172:errorcluster)  [unwired: 5 in, 1 out]
          }
        }
      }
      frame "Load Settings" {
        w179 = T11 {"Command"=enum."Fixed Range", "Data"=variant}  # Consumer Control
        n93 = call "Read Settings File.vi"("error in"=w182, "Cluster in"=w176) -> ("error out"=w175:errorcluster, "status"=w180:bool, "Cluster out"=w183:T21)  [unwired: 7 in]
        n94 = case shown="False" w180 {
          tunnel: w183 -> [w202 _]
          frame False {
            n95 = Unbundle(w202) -> ("Supply Voltage [Vdc]"=w201:sgl, "Max Supply Current [Idc]"=w200:sgl, "Settling Delay"=w199:dbl, "Temp Criteria"=w196:sgl, "Voltage Steps [Vrms]"=w197:sgl[], "User Notes"=w198:string, "Config Wave File Path"=w195:path, "Config Voltage [Vrms]"=w194:sgl, "Channel Configuration List"=w193:T3, "User Gains"=w192:T1, "Gains"=w191:T1, "Gain Array"=w190:T6, "Wave File Path 1"=w189:path, "Wave File Path 2"=w188:path, "Wave File Path 3"=w187:path, "Wave File Path 4"=w186:path, "Range"=w184:bool, "CF"=w185:bool)
            n96 = local write "Supply Volts"(w201) -> ()
            n97 = local write "Supply Amps"(w200) -> ()
            n98 = local write "Settling Delay"(w199) -> ()
            n99 = local write "Voltage Steps"(w197) -> ()
            n100 = local write "User Notes"(w198) -> ()
            n101 = local write "Data File"(w195) -> ()
            n102 = local write "Config Voltage"(w194) -> ()
            n103 = local write "Channel List"(w193) -> ()
            n104 = local write "User Gains"(w192) -> ()
            n105 = local write "Gain Averages"(w191) -> ()
            n106 = local write "Gain Array"(w190) -> ()
            n107 = local write "Wave File 1"(w189) -> ()
            n108 = local write "Wave File 2"(w188) -> ()
            n109 = local write "Wave File 3"(w187) -> ()
            n110 = local write "Wave File 4"(w186) -> ()
            n111 = local write "Range"(w184) -> ()
            n112 = local write "Crest Factor"(w185) -> ()
            n113 = local write "Temp Criteria"(w196) -> ()
          }
          frame True {
            n114 = One Button Dialog(message="An error occurred while loading Settings File.") -> ()  [unwired: 1 in, 1 out]
          }
        }
        n115 = Enqueue Element(queue=w178, element=w179, error in (no error)=w175) -> (queue out=w177:refnum<queue>, error out=w174:errorcluster)  [unwired: 1 in, 1 out]
      }
      frame "Power Test" {
        w206 = FALSE ("Visible")
        w209 = TRUE ("Visible")
        w217 = TRUE ("Visible")
        n116 = property on="Home" class="Bool"(error in=w221, "Visible"=w217) -> (error out=w219:errorcluster)  [unwired: 1 in, 1 out]
        n117 = local read "Range"() -> (w216:bool)
        n118 = property on="Run Test" class="Bool"(error in=w219, "Visible"=w217) -> (error out=w218:errorcluster)  [unwired: 1 in, 1 out]
        n119 = case shown="False" w216 {
          tunnel: w218 -> [w227 w228]
          tunnel: [w226 w228] -> w213
          tunnel: w217 -> [w225 _]
          frame False {
            n120 = property on="User Gains" class="Clust (strict)"(error in=w227, "Visible"=w225) -> (error out=w226:errorcluster)  [unwired: 1 in, 1 out]
          }
          frame True {
          }
        }
        n121 = property on="Power Graph" class="WFGraph (strict)"(error in=w213, "Visible"=w209) -> (error out=w215:errorcluster)  [unwired: 1 in, 1 out]
        n122 = property on="Heat" class="DigNum (strict)"(error in=w215, "Visible"=w209) -> (error out=w214:errorcluster)  [unwired: 1 in, 1 out]
        n123 = property on="Delay Countdown" class="DigNum (strict)"(error in=w214, "Visible"=w209) -> (error out=w204:errorcluster)  [unwired: 1 in, 1 out]
        n124 = property on="Total" class="DigNum (strict)"(error in=w204, "Visible"=w209) -> (error out=w211:errorcluster)  [unwired: 1 in, 1 out]
        n125 = property on="Current" class="DigNum (strict)"(error in=w211, "Visible"=w209) -> (error out=w210:errorcluster)  [unwired: 1 in, 1 out]
        n126 = property on="P Scale" class="Bool"(error in=w210, "Visible"=w209) -> (error out=w212:errorcluster)  [unwired: 1 in, 1 out]
        n127 = property on="Temp" class="Clust (strict)"(error in=w212, "Visible"=w206) -> (error out=w205:errorcluster)  [unwired: 1 in, 1 out]
        n128 = property on="Manual Warning" class="Bool"(error in=w205, "Visible"=w206, "DisabledEnum"=T12."Disabled" ("Disabled")) -> (error out=w208:errorcluster)  [unwired: 1 in, 1 out]
        n129 = property on="Tab Control" class="TabCtl (strict)"(error in=w208, "Value"=Functions_Tab."Power Test" ("Tab Control")) -> (error out=w223:errorcluster)  [unwired: 1 in, 1 out]
      }
      frame "Power Test M" {
        w231 = TRUE ("Visible")
        w234 = FALSE ("Visible")
        w242 = TRUE ("Visible")
        n130 = property on="Home" class="Bool"(error in=w246, "Visible"=w242) -> (error out=w244:errorcluster)  [unwired: 1 in, 1 out]
        n131 = local read "Range"() -> (w241:bool)
        n132 = property on="Run Test" class="Bool"(error in=w244, "Visible"=w242) -> (error out=w243:errorcluster)  [unwired: 1 in, 1 out]
        n133 = case shown="False" w241 {
          tunnel: w243 -> [w252 w253]
          tunnel: [w251 w253] -> w238
          tunnel: w242 -> [w250 _]
          frame False {
            n134 = property on="User Gains" class="Clust (strict)"(error in=w252, "Visible"=w250) -> (error out=w251:errorcluster)  [unwired: 1 in, 1 out]
          }
          frame True {
          }
        }
        n135 = property on="Power Graph" class="WFGraph (strict)"(error in=w238, "Visible"=w234) -> (error out=w240:errorcluster)  [unwired: 1 in, 1 out]
        n136 = property on="Heat" class="DigNum (strict)"(error in=w240, "Visible"=w234) -> (error out=w239:errorcluster)  [unwired: 1 in, 1 out]
        n137 = property on="Delay Countdown" class="DigNum (strict)"(error in=w239, "Visible"=w234) -> (error out=w229:errorcluster)  [unwired: 1 in, 1 out]
        n138 = property on="Total" class="DigNum (strict)"(error in=w229, "Visible"=w234) -> (error out=w236:errorcluster)  [unwired: 1 in, 1 out]
        n139 = property on="Current" class="DigNum (strict)"(error in=w236, "Visible"=w234) -> (error out=w235:errorcluster)  [unwired: 1 in, 1 out]
        n140 = property on="P Scale" class="Bool"(error in=w235, "Visible"=w234) -> (error out=w237:errorcluster)  [unwired: 1 in, 1 out]
        n141 = property on="Temp" class="Clust (strict)"(error in=w237, "Visible"=w231) -> (error out=w230:errorcluster)  [unwired: 1 in, 1 out]
        n142 = property on="Manual Warning" class="Bool"(error in=w230, "Visible"=w231, "DisabledEnum"=T12."Disabled" ("Disabled")) -> (error out=w233:errorcluster)  [unwired: 1 in, 1 out]
        n143 = property on="Tab Control" class="TabCtl (strict)"(error in=w233, "Value"=Functions_Tab."Power Test" ("Tab Control")) -> (error out=w248:errorcluster)  [unwired: 1 in, 1 out]
      }
      frame "Run Configuration" {
        w262 = FALSE ("Visible")
        n144 = property on="Run Configuration" class="Bool"(error in=w263, "Visible"=w262) -> (error out=w265:errorcluster)  [unwired: 1 in, 1 out]
        n145 = property on="Home" class="Bool"(error in=w265, "Visible"=w262) -> (error out=w261:errorcluster)  [unwired: 1 in, 1 out]
        n146 = Not(x=w262) -> (.not. x?=w264:bool)
        n147 = property on="Abort" class="Bool"(error in=w261, "Visible"=w264) -> (error out=w254:errorcluster)  [unwired: 1 in, 1 out]
        n148 = for {
          tunnel: w260 -> [w276]
          tunnel: w259 -> [w274]
          tunnel: dbl[] [10.0, 1.0] ("WT1800 Averages Out") -> [w272] mode=indexing
          shift-right: [w275] -> _
          shift-left: T1 {"Gain 1"=0.0, "Gain 2"=0.0, "Gain 3"=0.0, "Gain 4"=0.0, "Gain 5"=0.0, "Gain 6"=0.0} ("Gain Averages") -> [w273]
          shift-right: [w271] -> _
          shift-left: FALSE -> [w270]
          shift-right: [w269] -> w256
          shift-left: w254 -> [w268]
          n149 = case shown="False" w270 {
            selector: w270 -> [_ w374]
            tunnel: w276 -> [w319 _]
            tunnel: [w301 w373] -> w269
            tunnel: [w295 w375] -> w275
            tunnel: w274 -> [w294 _]
            tunnel: w273 -> [w292 w375]
            tunnel: w272 -> [w281 _]
            tunnel: [w278 w374] -> w271
            tunnel: w268 -> [w277 w373]
            frame False {
              w287 = FALSE ("Check EQ")
              w307 = sgl[][] [] ("WT1800 Averages Out")
              w306 = TRUE ("Reset Delay Clock")
              w314 = 6 ("Number of Elements")
              n150 = Bundle By Name(cluster=w294, "User Gains"=w292) -> (w293:T19)
              n151 = call "Read INI.vi"("Settings Cluster In"=w293, "Error In"=w277, "Command"=w319) -> ("Functions To Retreive"=w297:string[], "DSA Sampling Rate [Hz]"=w284:dbl, "WT1800 Instruments"=w322:refnum<visa-resource-name>[], "Update Rate [Seconds]"=w283:dbl, "Config Voltage [Vrms]"=w279:dbl, "DC Power Supply"=w291:refnum<visa-resource-name>, "DSA Input Channels"=w321:tag[], "DSA Output Channels"=w320:tag[], "Settings Cluster Out"=w290:T21, "Wave Generator Cluster Out"=w303:T22, "Error Out"=w289:errorcluster)  [unwired: 4 in, 2 out]
              n152 = call "Configure DC Power Supply.vi"("DC Power Supply In"=w291, "Error In"=w289, "Settings Cluster"=w290) -> ("error out"=w288:errorcluster)  [unwired: 15 in, 1 out]
              n153 = Multiply(x=w281, y=w279) -> (x*y=w296:dbl)
              n154 = Divide(x=w279, y=w281) -> (x/y=w280:dbl)
              n155 = Array Size(array=w297) -> (size(s)=w312:i32)
              n156 = call "WT1800 Configure Instruments.vi"("WT1800 Instruments In"=w322, "Check EQ"=w287, "Auto Range"=w287, "Channel Config"=TRUE, "Settings Cluster In"=w290, "Update Rate (50ms)"=w283, "Error In"=w288, "Voltage Step"=w296, "Fixed Range"=FALSE) -> ("WT1800 Instruments Out"=w316:refnum<visa-resource-name>[], "error out"=w304:errorcluster)  [unwired: 5 in]
              n157 = call "WT1800 Build Function Name List.vi"("Functions To Retreive"=w297, "Number of Channels"=w314) -> ("Array out"=w311:string[])  [unwired: 9 in]
              n158 = call "DSA Configure AI and AO.vi"("Input  Physical Channel"=w321, "Output Physical Channel"=w320, "Settings Cluster"=w290, "Wave Generator Cluster"=w303, "Sampling Rate [Hz]"=w284, "Error In"=w304, "Voltage Step"=w280, "Block Lenght (50ms)"=w283) -> ("Waveform"=w302:waveform(dbl)[][], "samples per channel"=w282:i32, "AI Task ID Out"=w318:refnum<k21>, "AO Task ID Out"=w317:refnum<k21>[], "Waveform Duration"=w309:dbl, "Error out"=w308:errorcluster)  [unwired: 4 in, 2 out]
              n159 = while {
                tunnel: w314 -> [w356]
                tunnel: w312 -> [w364]
                shift-right: [w366] -> _
                shift-left: w307 -> [w368]
                shift-right: [w335] -> _
                shift-left: w307 -> [w365]
                tunnel: 3 ("Channel Group") -> [w327]
                tunnel: w311 -> [w332]
                tunnel: w308 -> [w338]
                shift-right: [w357] -> _
                shift-left: 1 ("Iteration Count") -> [w355]
                tunnel: [w330] -> w310
                shift-right: [w370] -> _
                shift-left: w318 -> [w359]
                shift-right: [w369] -> _
                shift-left: w317 -> [w360]
                shift-right: [w358] -> _
                shift-left: w316 -> [w329]
                tunnel: [w350] -> w300
                shift-right: [w340] -> _
                shift-left: w306 -> [w352]
                tunnel: [w344] -> w278
                tunnel: w309 -> [w353]
                shift-right: [w339] -> _
                shift-left: w306 -> [w351]
                tunnel: [w349] -> w299
                tunnel: w302 -> [w347]
                shift-right: [w340] -> _
                shift-left: FALSE ("Step Delay Time has Elapsed Out") -> [w341]
                tunnel: w304 -> [w337]
                tunnel: w290 -> [w336]
                tunnel: w282 -> [w323]
                stop <- w354 stop-if-true
                n160 = call "DSA Step Delay and Waveform Reload.vi"("AI Task ID In"=w359, "AO Task ID In"=w360, "Settings Cluster"=w336, "Waveform Duration"=w353, "error in"=w338, "AO Waveform"=w347, "Step Delay Time has Elapsed In"=w341, "WT1800 Instruments"=w329, "Reset Delay Clock In"=w352, "Reset Test Clock In"=w351) -> ("Test Count Down"=→"Test Countdown 2":dbl, "Reset Test Clock Out"=w339:bool, "AI Task ID Out"=w362:refnum<k21>, "AO Task ID Out"=w361:refnum<k21>[], "Step Delay Time has Elapsed Out"=w340:bool, "Test Time has Elapsed Out"=w328:bool, "error out"=w363:errorcluster)  [unwired: 2 in, 1 out]
                n161 = Or(x=w328, y="Abort") -> (x .or. y?=w343:bool)
                n162 = call "DSA Measure Signal Amplitude and Levels.vi"("AI Task ID In"=w362, "AO Task ID In"=w361, "Step Delay Time has Elapsed"=w340, "Test Time has Elapsed"=w328, "error in"=w363, "samples per channel"=w323) -> ("Load Data"=w346:bool, "Task ID Cluster"=w371:T23, "DSA Measurements Array"=w334:sgl[][], "error out"=w325:errorcluster)  [unwired: 7 in, 3 out]
                n163 = call "WT1800 Read Measurements.vi"("WT1800 Instruments In"=w329, "WT1800 Channels per Instrument"=w356, "WT1800 Channel Group"=w327, "Number of Functions"=w364, "Desired Functions"=w332, "error in"=w337, "Step Delay Time has Elapsed"=w346) -> ("WT1800 Instruments Out"=w372:refnum<visa-resource-name>[], "WT1800 Measurements"=w333:sgl[][], "error out"=w348:errorcluster)  [unwired: 4 in, 2 out]
                n164 = call "Running Average.vi"("Load Data"=w346, "Iteration Count In"=w355, "DSA Measurements In"=w334, "WT1800 Measurements In"=w333, "DSA Averages In"=w365, "WT1800 Averages In"=w368) -> ("DSA Averages Out"=w335:sgl[][], "WT1800 Averages Out"=w366:sgl[][], "Iteration Count Out"=w357:i32)  [unwired: 3 in]
                n165 = call "Bundle Measurement Averages.vi"("WT1800 Channel Group"=w327, "WT1800 Measurements"=w366, "DSA Measurements"=w335, "WT1800 Channels per Instrument"=w356, "Number of Functions"=w364) -> ("WT1800 Averages"=w349:T8, "DSA Averages"=w350:T18)  [unwired: 8 in, 1 out]
                n166 = call "WT1800 Close Instruments.vi"("WT1800 Instruments In"=w372, "Buffer Complete In"=w343, "error in"=w348, "DSA Errors In"=w325) -> ("WT1800 Instruments Out"=w358:refnum<visa-resource-name>[], "Buffer Complete Out"=w326:bool, "error out"=w324:errorcluster)  [unwired: 9 in]
                n167 = call "DSA Stop AI and AO.vi"("Task ID Cluster"=w371, "error in"=w325, "Buffer Complete"=w326, "WT Errors In"=w324) -> ("AI Task ID Out"=w370:refnum<k21>, "AO Task ID Out"=w369:refnum<k21>[], "errors out"=w331:errorcluster)  [unwired: 13 in]
                n168 = Merge Errors(w324, w331) -> (w330:errorcluster)
                n169 = Unbundle By Name(w330) -> ("status"=w367:bool)
                n170 = Or(x=w367, y="Abort") -> (x .or. y?=w344:bool)
                n171 = Or(x=w343, y=w344) -> (x .or. y?=w354:bool)
              }
              n172 = call "Calculate Gains.vi"("DSA Averages"=w300, "WT1800 Averages"=w299, "error in"=w310, "Error or Abort"=w278, "Settings Cluster"=w290) -> ("Gain Averages"=w295:T1, "Gain Array"=→"Gain Array":T6, "error out"=w301:errorcluster)  [unwired: 6 in, 2 out]
              "Gain Averages" <- w295
              n173 = local write "User Gains"(w295) -> ()
            }
            frame True {
            }
          }
        }
        n174 = flat-sequence {
          tunnel: w264 -> [w378]
          tunnel: w256 -> [_]
          tunnel: w254 -> [w377]
          frame #0 {
            n175 = property on="Run Configuration" class="Bool"(error in=w377, "Visible"=w378) -> (error out=w379:errorcluster)  [unwired: 1 in, 1 out]
            n176 = property on="Home" class="Bool"(error in=w379, "Visible"=w378) -> (error out=w376:errorcluster)  [unwired: 1 in, 1 out]
            n177 = Not(x=w378) -> (.not. x?=w380:bool)
            n178 = property on="Abort" class="Bool"(error in=w376, "Visible"=w380) -> ()  [unwired: 1 in, 2 out]
          }
        }
      }
      frame "Run Test" {
        w407 = FALSE ("Visible")
        w402 = sgl[][] [] ("Graph")
        n179 = local read "Crest Factor"() -> (w388:bool)
        n180 = local read "Range"() -> (w398:bool)
        n181 = property on="Manual Warning" class="Bool"(error in=w383) -> (error out=w385:errorcluster, "Visible"=w381:bool)  [unwired: 1 in, 1 out]
        n182 = property on="Manual Warning" class="Bool"(error in=w385, "Blinking"=w381) -> (error out=w382:errorcluster)  [unwired: 1 in, 1 out]
        n183 = property on="Run Test" class="Bool"(error in=w382, "Visible"=w407) -> (error out=w411:errorcluster)  [unwired: 1 in, 1 out]
        n184 = property on="Home" class="Bool"(error in=w411, "Visible"=w407) -> (error out=w406:errorcluster)  [unwired: 1 in, 1 out]
        n185 = Not(x=w407) -> (.not. x?=w410:bool)
        n186 = property on="Stop" class="Bool"(error in=w406, "Visible"=w410) -> (error out=w384:errorcluster)  [unwired: 1 in, 1 out]
        n187 = call "Read INI.vi"("Settings Cluster In"=w404, "Run Mode (Manual = True)"=w381, "Error In"=w384, "Command"=w405) -> ("Functions To Retreive"=w414:string[], "DSA Sampling Rate [Hz]"=w386:dbl, "WT1800 Instruments"=w415:refnum<visa-resource-name>[], "Update Rate [Seconds]"=w416:dbl, "Voltage Steps [Vrms]"=w397:dbl[], "DC Power Supply"=w401:refnum<visa-resource-name>, "DSA Input Channels"=w409:tag[], "DSA Output Channels"=w408:tag[], "Settings Cluster Out"=w393:T21, "Wave Generator Cluster Out"=w417:T22, "Error Out"=w400:errorcluster)  [unwired: 3 in, 2 out]
        n188 = Array Size(array=w397) -> (size(s)=w389:i32)
        "Total" <- w389
        n189 = call "Configure DC Power Supply.vi"("DC Power Supply In"=w401, "Error In"=w400, "Settings Cluster"=w393) -> ("error out"=w399:errorcluster)  [unwired: 15 in, 1 out]
        n190 = for {
          tunnel: w409 -> [w450]
          tunnel: w408 -> [w449]
          tunnel: w416 -> [w448]
          tunnel: w415 -> [w451]
          tunnel: w397 -> [w445] mode=indexing
          tunnel: w414 -> [w447]
          shift-right: [w446] -> w392
          shift-left: w399 -> [w444]
          shift-right: [w443] -> w390
          shift-left: FALSE -> [w442]
          shift-right: [w441] -> _
          shift-left: w402 -> [w440]
          tunnel: w393 -> [w439]
          tunnel: w417 -> [w438]
          tunnel: T13[][] [] -> [w437]
          tunnel: [w436] -> w391 mode=indexing
          tunnel: w402 -> [w435]
          tunnel: [w434] -> w394
          tunnel: [w433] -> w395
          tunnel: [w432] -> w396
          tunnel: w398 -> [w431]
          tunnel: w389 -> [w430]
          tunnel: w388 -> [w428]
          tunnel: w386 -> [w427]
          tunnel: w381 -> [w426]
          i -> [w429]
          n191 = case shown="False" w442 {
            selector: w442 -> [_ w681]
            tunnel: w451 -> [w474 _]
            tunnel: w450 -> [w473 _]
            tunnel: w449 -> [w472 _]
            tunnel: w448 -> [w467 _]
            tunnel: w447 -> [w471 _]
            tunnel: [w470 w682] -> w446
            tunnel: w444 -> [w475 w682]
            tunnel: w445 -> [w468 _]
            tunnel: [w464 w681] -> w443
            tunnel: [w465 w680] -> w441
            tunnel: w440 -> [w476 w680]
            tunnel: w439 -> [w466 _]
            tunnel: w438 -> [w469 _]
            tunnel: w437 -> [w463 _]
            tunnel: [w462 T15 {"Heat"=0.0, "WT1800 Functions"=[], "WT1800 Averages"=[], "WT1800 Measurements"=[], "DSA Functions"=[], "DSA Averages"=[], "DSA Measurements"=[], "Initial Time Stamp"=timestamp(0 s since 1904-01-01), "Final Time Stamp"=timestamp(0 s since 1904-01-01), "Temperature Data"=[]} ("Datalog Cluster")] -> w436
            tunnel: w435 -> [w461 _]
            tunnel: [w460 _] -> w434
            tunnel: [w459 _] -> w433
            tunnel: [w458 _] -> w432
            tunnel: w431 -> [w457 _]
            tunnel: w430 -> [w456 _]
            tunnel: w429 -> [w455 _]
            tunnel: w428 -> [w454 _]
            tunnel: w427 -> [w453 _]
            tunnel: w426 -> [w452 _]
            frame False {
              n192 = stacked-sequence {
                tunnel: w476 -> [_ w518 _ _ _]
                tunnel: w475 -> [_ w528 _ _ _]
                tunnel: w474 -> [_ w537 _ _ _]
                tunnel: w473 -> [_ w541 _ _ _]
                tunnel: w472 -> [_ w540 _ _ _]
                tunnel: w471 -> [_ w529 _ _ _]
                tunnel: [_ w514 _ _ _] -> w470
                tunnel: w469 -> [_ w531 _ _ _]
                tunnel: w468 -> [_ w522 _ _ _]
                tunnel: w467 -> [_ w495 _ _ _]
                tunnel: w466 -> [_ w534 _ _ _]
                tunnel: [_ w517 _ _ _] -> w465
                tunnel: [_ w496 _ _ _] -> w464
                tunnel: w463 -> [_ w519 _ _ _]
                tunnel: [_ w505 _ _ _] -> w462
                tunnel: w461 -> [_ w500 _ _ _]
                tunnel: [_ _ _ _ w654] -> w460
                tunnel: [_ _ _ _ w653] -> w459
                tunnel: [_ _ _ _ w651] -> w458
                tunnel: w457 -> [w481 w501 _ _ w646]
                tunnel: w456 -> [_ _ _ _ w649]
                tunnel: w455 -> [w479 _ _ _ w648]
                tunnel: w454 -> [_ w499 _ _ _]
                tunnel: w453 -> [_ w498 _ _ _]
                tunnel: w452 -> [_ w493 _ _ _]
                frame #0 {
                  n193 = Increment(x=w479) -> (x+1=→"Current":i32)
                  n194 = Equal To 0?(x=w479) -> (x = 0?=w480:bool)
                  n195 = case shown="True" w480 {
                    tunnel: w481 -> [_ w482]
                    frame False {
                    }
                    frame True {
                      n196 = case shown="True" w482 {
                        selector: w482 -> [_ w483]
                        frame False {
                        }
                        frame True {
                          n197 = stacked-sequence {
                            tunnel: w483 -> [w486 _ _ w490]
                            frame #0 {
                              n198 = Not(x=w486) -> (.not. x?=w484:bool)
                              n199 = property on="Next Button" class="Bool (strict)"("Visible"=w486, "Key Focus"=w486, "Blinking"=w486) -> ()  [unwired: 2 in, 2 out]
                              n200 = property on="Range" class="Bool (strict)"("Visible"=w484) -> ()  [unwired: 2 in, 2 out]
                              n201 = property on="Tab Control" class="TabCtl (strict)"("Value"=Functions_Tab."Channel Configuration" ("Tab Control")) -> ()  [unwired: 2 in, 2 out]
                            }
                            frame #1 {
                              n202 = while {
                                stop <- w487 stop-if-true
                                n203 = local read "Next Button"() -> (w487:bool)
                                n204 = Wait (ms)(milliseconds to wait=u32 50) -> ()  [unwired: 1 out]
                              }
                            }
                            frame #2 {
                              n205 = local write "Next Button"(FALSE ("Next Button")) -> ()
                            }
                            frame #3 {
                              n206 = Not(x=w490) -> (.not. x?=w492:bool)
                              n207 = property on="Next Button" class="Bool (strict)"("Visible"=w492, "Key Focus"=w492, "Blinking"=w492) -> ()  [unwired: 2 in, 2 out]
                              n208 = property on="Range" class="Bool (strict)"("Visible"=w490) -> ()  [unwired: 2 in, 2 out]
                              n209 = property on="Tab Control" class="TabCtl (strict)"("Value"=Functions_Tab."Power Test" ("Tab Control")) -> ()  [unwired: 2 in, 2 out]
                            }
                          }
                        }
                      }
                    }
                  }
                  "Temp" <- T14 {"1"=0.0, "2"=0.0, "3"=0.0, "4"=0.0, "5"=0.0, "6"=0.0, "7"=0.0, "8"=0.0, "9"=0.0, "10"=0.0, "11"=0.0, "12"=0.0, "13"=0.0, "14"=0.0, "15"=0.0, "16"=0.0, "17"=0.0, "18"=0.0, "19"=0.0, "20"=0.0, "21"=0.0, "22"=0.0, "23"=0.0, "24"=0.0, "25"=0.0, "26"=0.0, "27"=0.0, "28"=0.0, "29"=0.0, "30"=0.0, "31"=0.0, "32"=0.0} ("Temp")
                }
                frame #1 {
                  w504 = FALSE ("Check EQ")
                  w521 = TRUE ("Reset Delay Clock")
                  w535 = 6 ("Number of Elements")
                  n210 = Array Size(array=w529) -> (size(s)=w532:i32)
                  n211 = local read "Channel List"() -> (w502:T3)
                  n212 = call "WT1800 Configure Instruments.vi"("WT1800 Instruments In"=w537, "Check EQ"=w504, "Auto Range"=w504, "Channel Configuration List"=w502, "Channel Config"=w504, "Settings Cluster In"=w534, "Update Rate (50ms)"=w495, "Error In"=w528, "Voltage Step"=w522, "Fixed Range"=w501, "Crest Factor"=w499) -> ("WT1800 Instruments Out"=w536:refnum<visa-resource-name>[], "error out"=w523:errorcluster)  [unwired: 3 in]
                  n213 = call "WT1800 Build Function Name List.vi"("Functions To Retreive"=w529, "Number of Channels"=w535) -> ("Array out"=w530:string[])  [unwired: 9 in]
                  n214 = call "DSA Configure AI and AO.vi"("Input  Physical Channel"=w541, "Output Physical Channel"=w540, "Settings Cluster"=w534, "Wave Generator Cluster"=w531, "Sampling Rate [Hz]"=w498, "Error In"=w523, "Voltage Step"=w522, "Run Mode (Manual = True)"=w493, "Block Lenght (50ms)"=w495) -> ("Waveform"=w515:waveform(dbl)[][], "samples per channel"=w494:i32, "AI Task ID Out"=w539:refnum<k21>, "AO Task ID Out"=w538:refnum<k21>[], "Waveform Duration"=w526:dbl, "Step Delay"=w525:dbl, "Error out"=w524:errorcluster)  [unwired: 3 in, 1 out]
                  n215 = while {
                    tunnel: w535 -> [w591]
                    tunnel: w532 -> [w600]
                    shift-right: [w602] -> _
                    shift-left: w500 -> [w604]
                    shift-right: [w562] -> _
                    shift-left: w500 -> [w601]
                    tunnel: 3 ("Channel Group") -> [w554]
                    tunnel: w530 -> [w561]
                    tunnel: w524 -> [w569]
                    shift-right: [w592] -> _
                    shift-left: 1 ("Iteration Count") -> [w590]
                    tunnel: [w556] -> w527
                    shift-right: [w606] -> _
                    shift-left: w539 -> [w595]
                    shift-right: [w605] -> _
                    shift-left: w538 -> [w596]
                    shift-right: [w594] -> _
                    shift-left: w536 -> [w560]
                    shift-right: [w593] -> w510
                    shift-left: w519 -> [w608]
                    tunnel: [w583] -> w509
                    shift-right: [w572] -> _
                    shift-left: w521 -> [w586]
                    tunnel: [w574] -> w497
                    tunnel: w526 -> [w588]
                    tunnel: w525 -> [w587]
                    shift-right: [w571] -> _
                    shift-left: w521 -> [w585]
                    tunnel: [w581] -> w508
                    shift-right: [w584] -> w511
                    shift-left: w519 -> [w607]
                    tunnel: w515 -> [w577]
                    shift-right: [w572] -> _
                    shift-left: FALSE ("Reset Delay Clock") -> [w573]
                    tunnel: w534 -> [w570]
                    tunnel: w523 -> [w568]
                    shift-right: [w566] -> w512
                    shift-left: _ -> [w564]
                    shift-right: [w565] -> w513
                    shift-left: _ -> [w563]
                    shift-right: [w543] -> w503
                    shift-left: w500 -> [w544]
                    tunnel: w494 -> [w546]
                    tunnel: w493 -> [w545]
                    stop <- w589 stop-if-true
                    n216 = call "DSA Step Delay and Waveform Reload.vi"("AI Task ID In"=w595, "AO Task ID In"=w596, "Settings Cluster"=w570, "Waveform Duration"=w588, "Step Delay"=w587, "error in"=w569, "AO Waveform"=w577, "Step Delay Time has Elapsed In"=w573, "WT1800 Instruments"=w560, "Reset Delay Clock In"=w586, "Reset Test Clock In"=w585) -> ("Step Delay Count Down"=→"Delay Countdown":dbl, "Test Count Down"=→"Test Countdown":dbl, "Reset Test Clock Out"=w571:bool, "AI Task ID Out"=w598:refnum<k21>, "AO Task ID Out"=w597:refnum<k21>[], "Step Delay Time has Elapsed Out"=w572:bool, "Test Time has Elapsed Out"=w553:bool, "error out"=w599:errorcluster)  [unwired: 1 in]
                    n217 = Or(x=w553, y="Stop") -> (x .or. y?=w555:bool)
                    n218 = call "DSA Measure Signal Amplitude and Levels.vi"("AI Task ID In"=w598, "AO Task ID In"=w597, "Step Delay Time has Elapsed"=w572, "Test Time has Elapsed"=w553, "error in"=w599, "samples per channel"=w546, "Run Mode (Manual = True)"=w545) -> ("Load Data"=w576:bool, "Task ID Cluster"=w609:T23, "DSA Measurements Array"=w558:sgl[][], "DSA Measurements"=w548:T18, "DSA Functions"=w547:T17, "Temperature Data"=w542:sgl[], "error out"=w550:errorcluster)  [unwired: 6 in]
                    n219 = call "WT1800 Read Measurements.vi"("WT1800 Instruments In"=w560, "WT1800 Channels per Instrument"=w591, "WT1800 Channel Group"=w554, "Number of Functions"=w600, "Desired Functions"=w561, "error in"=w568, "Step Delay Time has Elapsed"=w576) -> ("WT1800 Instruments Out"=w610:refnum<visa-resource-name>[], 6:"WT1800 Measurements"=w559:sgl[][], 8:"WT1800 Measurements"=w582:T8, "WT1800 Functions"=w567:T16, "error out"=w578:errorcluster)  [unwired: 4 in]
                    n220 = call "Running Average.vi"("Load Data"=w576, "Iteration Count In"=w590, "DSA Measurements In"=w558, "WT1800 Measurements In"=w559, "DSA Averages In"=w601, "WT1800 Averages In"=w604) -> ("DSA Averages Out"=w562:sgl[][], "WT1800 Averages Out"=w602:sgl[][], "Iteration Count Out"=w592:i32)  [unwired: 3 in]
                    n221 = Array To Cluster(array=w542) -> (cluster=w549:T24)
                    n222 = call "Bundle Measurement Averages.vi"("WT1800 Channel Group"=w554, "WT1800 Measurements"=w602, "DSA Measurements"=w562, "WT1800 Channels per Instrument"=w591, "Number of Functions"=w600) -> ("WT1800 Averages"=w581:T8, "DSA Averages"=w583:T18)  [unwired: 8 in, 1 out]
                    n223 = call "WT1800 Close Instruments.vi"("WT1800 Instruments In"=w610, "Buffer Complete In"=w555, "error in"=w578, "DSA Errors In"=w550) -> ("WT1800 Instruments Out"=w594:refnum<visa-resource-name>[], "Buffer Complete Out"=w552:bool, "error out"=w551:errorcluster)  [unwired: 9 in]
                    n224 = call "DSA Stop AI and AO.vi"("Task ID Cluster"=w609, "error in"=w550, "Buffer Complete"=w552, "WT Errors In"=w551) -> ("AI Task ID Out"=w606:refnum<k21>, "AO Task ID Out"=w605:refnum<k21>[], "errors out"=w557:errorcluster)  [unwired: 13 in]
                    n225 = local write "Temp"(w549) -> ()
                    n226 = Merge Errors(w551, w557) -> (w556:errorcluster)
                    n227 = case shown="True" w576 {
                      tunnel: w582 -> [_ w624]
                      tunnel: w608 -> [w615 w626]
                      tunnel: [w615 w625] -> w593
                      tunnel: w548 -> [_ w622]
                      tunnel: [w614 w621] -> w584
                      tunnel: w607 -> [w614 w623]
                      tunnel: [w613 w620] -> w566
                      tunnel: w567 -> [_ w620]
                      tunnel: [w612 w619] -> w565
                      tunnel: w547 -> [_ w619]
                      tunnel: w564 -> [w613 _]
                      tunnel: w563 -> [w612 _]
                      tunnel: [w611 w617] -> w543
                      tunnel: w544 -> [w611 w618]
                      tunnel: w542 -> [_ w616]
                      frame False {
                      }
                      frame True {
                        n228 = Build Array (concatenate)(w626, w624) -> (w625:T9[][])
                        n229 = Build Array (concatenate)(w623, w622) -> (w621:T13[][])
                        n230 = Build Array (concatenate)(w618, w616) -> (w617:sgl[][])
                      }
                    }
                    n231 = local write "WT1800"(w581) -> ()
                    n232 = Unbundle By Name(w556) -> ("status"=w603:bool)
                    n233 = Or(x=w603, y="Stop") -> (x .or. y?=w574:bool)
                    n234 = Or(x=w555, y=w574) -> (x .or. y?=w589:bool)
                  }
                  "WT1800" <- w508
                  n235 = call "Bundle Data Log.vi"("DSA Measurements"=w511, "WT1800 Measurements"=w510, "DSA Averages"=w509, "WT1800 Averages"=w508, "WT1800 Functions"=w512, "DSA Functions"=w513, "Temperature Data"=w503, "error in (no error)"=w527, "Error or Abort"=w497, "Run Mode (Manual = True)"=w493) -> ("Average Power + Heat"=w507:dbl[], "Heat"=→"Heat":dbl, "Datalog Cluster"=w505:T15, "Error or Abort Out"=w496:bool, "error out"=w514:errorcluster)  [unwired: 1 in]
                  n236 = Build Array (concatenate)(w518, w507) -> (w517:dbl[][])
                  "Power Graph" <- w517
                  "V Step" <- w522
                }
                frame #2 {
                  w627 = u8 1 ("X Scale.Scale Fit")
                  n237 = property on="Power Graph" class="WFGraph (strict)"("XScale.ScaleFit"=w627, "YScale.ScaleFit"=w627) -> ()  [unwired: 2 in, 2 out]
                }
                frame #3 {
                  n238 = property on="Power Graph" class="WFGraph (strict)"() -> ("YScale.Maximum"=w630:dbl, "YScale.Minimum"=w629:dbl)  [unwired: 2 in, 2 out]
                  n239 = Subtract(x=w630, y=w629) -> (x-y=w634:dbl)
                  n240 = Divide(x=w634, y=2.0) -> (x/y=w633:dbl)
                  n241 = Add(x=w633, y=w629) -> (x+y=w632:dbl)
                  n242 = Bundle(1000.0, w632) -> (w628:cluster{dbl, dbl})  [unwired: 1 in]
                  n243 = property on="Power Graph" class="WFGraph (strict)"("Cursor.Cursor Position"=w628) -> ()  [unwired: 2 in, 2 out]
                }
                frame #4 {
                  n244 = Increment(x=w648) -> (x+1=w650:i32)
                  n245 = Equal?(x=w649, y=w650) -> (x = y?=w647:bool)
                  n246 = Current VI's Path() -> (path=w642:path)
                  n247 = Strip Path(path=w642) -> (stripped path=w641:path)  [unwired: 1 out]
                  n248 = local read "Data File"() -> (w644:path)
                  n249 = Strip Path(path=w641) -> (stripped path=w639:path)  [unwired: 1 out]
                  n250 = Build Path(base path=w639, name or relative path="Data") -> (appended path=w638:path)
                  n251 = call <vilib>:"Is Path and Not Empty.vi"("path"=w644) -> ("Is Path and Not Empty?"=w645:bool)  [unwired: 4 in]
                  n252 = Select(t=w644, s=w645, f=path "C:/ASD_PowerPoint_TestData" ("Data File")) -> (s? t:f=w637:path)
                  n253 = Create Folder(path (use dialog)=w637) -> (created path=w636:path)  [unwired: 2 in, 2 out]
                  n254 = Build Path(base path=w636, name or relative path="EQ_Graph.jpg") -> (appended path=w654:path)
                  n255 = Build Path(base path=w636, name or relative path="Z_Graph.jpg") -> (appended path=w653:path)
                  n256 = case shown="True" w647 {
                    tunnel: w654 -> [_ w671]
                    tunnel: w653 -> [_ w670]
                    tunnel: w646 -> [w657 _]
                    frame False {
                      n257 = case shown="True" w657 {
                        selector: w657 -> [_ w658]
                        frame False {
                        }
                        frame True {
                          n258 = stacked-sequence {
                            tunnel: w658 -> [w661 _ _ w665]
                            frame #0 {
                              n259 = Not(x=w661) -> (.not. x?=w659:bool)
                              n260 = property on="Next Button" class="Bool (strict)"("Visible"=w661, "Key Focus"=w661, "Blinking"=w661) -> ()  [unwired: 2 in, 2 out]
                              n261 = property on="Range" class="Bool (strict)"("Visible"=w659) -> ()  [unwired: 2 in, 2 out]
                              n262 = property on="Tab Control" class="TabCtl (strict)"("Value"=Functions_Tab."Channel Configuration" ("Tab Control")) -> ()  [unwired: 2 in, 2 out]
                            }
                            frame #1 {
                              n263 = while {
                                stop <- "Next Button" stop-if-true
                                n264 = Wait (ms)(milliseconds to wait=u32 50) -> ()  [unwired: 1 out]
                              }
                            }
                            frame #2 {
                              n265 = local write "Next Button"(FALSE ("Next Button")) -> ()
                            }
                            frame #3 {
                              n266 = Not(x=w665) -> (.not. x?=w667:bool)
                              n267 = property on="Next Button" class="Bool (strict)"("Visible"=w667, "Key Focus"=w667, "Blinking"=w667) -> ()  [unwired: 2 in, 2 out]
                              n268 = property on="Range" class="Bool (strict)"("Visible"=w665) -> ()  [unwired: 2 in, 2 out]
                              n269 = property on="Tab Control" class="TabCtl (strict)"("Value"=Functions_Tab."Power Test" ("Tab Control")) -> ()  [unwired: 2 in, 2 out]
                            }
                          }
                        }
                      }
                    }
                    frame True {
                      w672 = 95 ("quality (80)")
                      w677 = u32 11844819
                      w678 = 24 ("Image Depth")
                      n270 = control-ref of="EQ Graph"() -> (w676:refnum<vi>)
                      n271 = control-ref of="Z Graph"() -> (w675:refnum<vi>)
                      n272 = invoke on="Invoke Node" class="XYGraph (strict)" method="Get Image"(reference=w676, "image depth"=w678, "bg color"=w677) -> ("image data"=w674:T25)  [unwired: 3 in, 5 out]
                      n273 = invoke on="Invoke Node" class="XYGraph (strict)" method="Get Image"(reference=w675, "image depth"=w678, "bg color"=w677) -> ("image data"=w673:T25)  [unwired: 3 in, 5 out]
                      n274 = call <vilib>:"Write JPEG File.vi"("quality (80)"=w672, "image data"=w674, "path to JPEG file"=w671) -> ("error out"=w669:errorcluster)  [unwired: 7 in, 1 out]
                      n275 = call <vilib>:"Write JPEG File.vi"("quality (80)"=w672, "error in (no error)"=w669, "image data"=w673, "path to JPEG file"=w670) -> ("error out"=w668:errorcluster)  [unwired: 6 in, 1 out]
                      n276 = call <vilib>:"Simple Error Handler.vi"("error in (no error)"=w668) -> ()  [unwired: 4 in, 5 out]
                    }
                  }
                  n277 = Build Path(base path=w638, name or relative path="ASD Template.xls") -> (appended path=w651:path)
                }
              }
            }
            frame True {
            }
          }
        }
        n278 = flat-sequence {
          tunnel: w410 -> [w423]
          tunnel: w392 -> [_]
          tunnel: w384 -> [w422]
          frame #0 {
            n279 = property on="Run Test" class="Bool"(error in=w422, "Visible"=w423) -> (error out=w424:errorcluster)  [unwired: 1 in, 1 out]
            n280 = property on="Home" class="Bool"(error in=w424, "Visible"=w423) -> (error out=w421:errorcluster)  [unwired: 1 in, 1 out]
            n281 = Not(x=w423) -> (.not. x?=w425:bool)
            n282 = property on="Stop" class="Bool"(error in=w421, "Visible"=w425) -> (error out=w420:errorcluster)  [unwired: 1 in, 1 out]
            n283 = property on="Manual Warning" class="Bool"(error in=w420, "Blinking"=FALSE) -> ()  [unwired: 1 in, 2 out]
          }
        }
        n284 = call "Excel Data Log 2.vi"("Channel Settings"=w393, "JPEG2 Path"=w394, "Cancel"=w390, "JPEG1 Path"=w395, "error in"=w392, "Datalog Cluster Array"=w391, "Template Path"=w396) -> ("error out"=w387:errorcluster)  [unwired: 4 in]
      }
      frame "Abort" {
      }
      frame "Run EQ" {
        w698 = TRUE  # Check EQ
        w699 = sgl[][] []
        w712 = FALSE ("Visible")
        n285 = local read "Crest Factor"() -> (w690:bool)
        n286 = local read "Range"() -> (w691:bool)
        n287 = property on="Run EQ Check" class="Bool"(error in=w716, "Visible"=w712) -> (error out=w718:errorcluster)  [unwired: 1 in, 1 out]
        n288 = property on="Home" class="Bool"(error in=w718, "Visible"=w712) -> (error out=w710:errorcluster)  [unwired: 1 in, 1 out]
        n289 = Not(x=w712) -> (.not. x?=w717:bool)
        n290 = property on="Abort 3" class="Bool"(error in=w710, "Visible"=w717) -> (error out=w711:errorcluster)  [unwired: 1 in, 1 out]
        n291 = call "Read INI.vi"("EQ Measurement Resolution"="Resolution", "Settings Cluster In"=w713, "Auto Range"="Auto Range", "Error In"=w711, "Command"=w709) -> ("Functions To Retreive"=w700:string[], "DSA Sampling Rate [Hz]"=w689:dbl, "WT1800 Instruments"=w720:refnum<visa-resource-name>[], "Update Rate [Seconds]"=w702:dbl, "EQ Check Wave Array"=w707:T22[], "Config Voltage [Vrms]"=w708:dbl, "DC Power Supply"=w693:refnum<visa-resource-name>, "DSA Input Channels"=w715:tag[], "DSA Output Channels"=w714:tag[], "Settings Cluster Out"=w694:T21, "Error Out"=w696:errorcluster)  [unwired: 2 in, 2 out]
        n292 = call "Configure DC Power Supply.vi"("DC Power Supply In"=w693, "Error In"=w696, "Settings Cluster"=w694) -> ("error out"=w695:errorcluster)  [unwired: 15 in, 1 out]
        n293 = call "WT1800 Configure Instruments.vi"("WT1800 Instruments In"=w720, "Check EQ"=w698, "Auto Range"="Auto Range", "Channel Config"=FALSE, "Settings Cluster In"=w694, "Update Rate (50ms)"=w702, "Error In"=w695, "Voltage Step"=w708, "Fixed Range"=w691, "Crest Factor"=w690) -> ("WT1800 Instruments Out"=w706:refnum<visa-resource-name>[], "error out"=w701:errorcluster)  [unwired: 4 in]
        n294 = for {
          tunnel: w694 -> [w743]
          tunnel: w700 -> [w742]
          tunnel: w715 -> [w741]
          tunnel: w714 -> [w740]
          tunnel: [w739] -> w687
          tunnel: w708 -> [w738]
          tunnel: w702 -> [w737]
          tunnel: w707 -> [w736] mode=indexing
          tunnel: w706 -> [w735]
          tunnel: w701 -> [w734]
          shift-right: [w733] -> _
          shift-left: FALSE -> [w724]
          shift-right: [w726] -> _
          shift-left: w699 -> [w730]
          shift-right: [w727] -> _
          shift-left: w699 -> [w731]
          shift-right: [w729] -> _
          shift-left: dbl[] [] -> [w732]
          tunnel: w701 -> [w728]
          tunnel: w699 -> [w725]
          tunnel: w689 -> [w723]
          tunnel: [w722] -> w688
          n295 = case shown="False" w724 {
            selector: w724 -> [_ w871]
            tunnel: w743 -> [w764 _]
            tunnel: w742 -> [w763 _]
            tunnel: w741 -> [w762 _]
            tunnel: w740 -> [w761 _]
            tunnel: [w760 errorcluster {"status"=FALSE, "code"=0, "source"=""} ("error out")] -> w739
            tunnel: w738 -> [w759 _]
            tunnel: w737 -> [w758 _]
            tunnel: w736 -> [w757 _]
            tunnel: w735 -> [w756 w870]
            tunnel: w734 -> [w755 _]
            tunnel: [w754 w871] -> w733
            tunnel: w732 -> [w753 w873]
            tunnel: w731 -> [w752 w874]
            tunnel: w730 -> [w751 w875]
            tunnel: [w750 w873] -> w729
            tunnel: w728 -> [w749 _]
            tunnel: [w748 w874] -> w727
            tunnel: [w747 w875] -> w726
            tunnel: w725 -> [w746 _]
            tunnel: w723 -> [w745 _]
            tunnel: [w744 w870] -> w722
            frame False {
              n296 = stacked-sequence {
                tunnel: w764 -> [w807 _ _]
                tunnel: w763 -> [w806 _ _]
                tunnel: w762 -> [w805 _ _]
                tunnel: w761 -> [w804 _ _]
                tunnel: [w803 _ _] -> w760
                tunnel: w759 -> [w802 _ _]
                tunnel: w758 -> [w767 _ _]
                tunnel: w757 -> [w801 _ _]
                tunnel: w756 -> [w800 _ _]
                tunnel: w755 -> [w799 _ _]
                tunnel: [w798 _ _] -> w754
                tunnel: w753 -> [w796 _ _]
                tunnel: w752 -> [w795 _ _]
                tunnel: w751 -> [w794 _ _]
                tunnel: [w790 _ _] -> w750
                tunnel: w749 -> [w793 _ _]
                tunnel: [w789 _ _] -> w748
                tunnel: [w788 _ _] -> w747
                tunnel: w746 -> [w785 _ _]
                tunnel: w745 -> [w768 _ _]
                tunnel: [w766 _ _] -> w744
                frame #0 {
                  w773 = TRUE ("Reset Delay Clock")
                  w781 = 6 ("Number of Elements")
                  n297 = Array Size(array=w806) -> (size(s)=w779:i32)
                  n298 = call "WT1800 Build Function Name List.vi"("Functions To Retreive"=w806, "Number of Channels"=w781) -> ("Array out"=w778:string[])  [unwired: 9 in]
                  n299 = call "DSA Configure AI and AO.vi"("Input  Physical Channel"=w805, "Output Physical Channel"=w804, "Settings Cluster"=w807, "Wave Generator Cluster"=w801, "Sampling Rate [Hz]"=w768, "Error In"=w799, "Voltage Step"=w802, "Block Lenght (50ms)"=w767) -> ("Waveform"=w774:waveform(dbl)[][], "samples per channel"=w765:i32, "AI Task ID Out"=w784:refnum<k21>, "AO Task ID Out"=w783:refnum<k21>[], "Waveform Duration"=w776:dbl, "Error out"=w775:errorcluster)  [unwired: 4 in, 2 out]
                  n300 = while {
                    tunnel: w781 -> [w836]
                    tunnel: w779 -> [w845]
                    shift-right: [w847] -> _
                    shift-left: w785 -> [w849]
                    shift-right: [w828] -> _
                    shift-left: w785 -> [w846]
                    tunnel: 3 ("Channel Group") -> [w829]
                    tunnel: w778 -> [w842]
                    tunnel: w775 -> [w816]
                    shift-right: [w837] -> _
                    shift-left: 1 ("Iteration Count") -> [_]
                    tunnel: [w814] -> w777
                    shift-right: [w851] -> _
                    shift-left: w784 -> [w838]
                    shift-right: [w850] -> _
                    shift-left: w783 -> [w839]
                    shift-right: [w810] -> w766
                    shift-left: w800 -> [w823]
                    tunnel: [w831] -> w771
                    shift-right: [w818] -> _
                    shift-left: w773 -> [w833]
                    tunnel: [w821] -> w798
                    tunnel: w776 -> [w834]
                    shift-right: [w817] -> _
                    shift-left: w773 -> [w832]
                    tunnel: [w827] -> w770
                    tunnel: w774 -> [w826]
                    shift-right: [w818] -> _
                    shift-left: FALSE ("Step Delay Time has Elapsed Out") -> [w820]
                    tunnel: w793 -> [w815]
                    tunnel: w765 -> [w808]
                    stop <- w835 stop-if-true
                    n301 = call "DSA Step Delay and Waveform Reload.vi"("AI Task ID In"=w838, "AO Task ID In"=w839, "Waveform Duration"=w834, "error in"=w816, "AO Waveform"=w826, "Step Delay Time has Elapsed In"=w820, "WT1800 Instruments"=w823, "Reset Delay Clock In"=w833, "Reset Test Clock In"=w832) -> ("Reset Test Clock Out"=w817:bool, "AI Task ID Out"=w841:refnum<k21>, "AO Task ID Out"=w840:refnum<k21>[], "Step Delay Time has Elapsed Out"=w818:bool, "Test Time has Elapsed Out"=w819:bool, "error out"=w843:errorcluster)  [unwired: 3 in, 2 out]
                    n302 = Or(x=w819, y="Abort 3") -> (x .or. y?=w809:bool)
                    n303 = call "DSA Measure Signal Amplitude and Levels.vi"("AI Task ID In"=w841, "AO Task ID In"=w840, "Step Delay Time has Elapsed"=w818, "Test Time has Elapsed"=w819, "error in"=w843, "samples per channel"=w808) -> ("Load Data"=w824:bool, "Task ID Cluster"=w852:T23, "DSA Measurements Array"=w830:sgl[][], "error out"=w812:errorcluster)  [unwired: 7 in, 3 out]
                    n304 = call "WT1800 Read Measurements.vi"("WT1800 Instruments In"=w823, "WT1800 Channels per Instrument"=w836, "WT1800 Channel Group"=w829, "Number of Functions"=w845, "Desired Functions"=w842, "error in"=w815, "Step Delay Time has Elapsed"=w824) -> ("WT1800 Instruments Out"=w810:refnum<visa-resource-name>[], "WT1800 Measurements"=w844:sgl[][], "error out"=w811:errorcluster)  [unwired: 4 in, 2 out]
                    n305 = call "Running Average.vi"("Load Data"=w824, "Iteration Count In"=1, "DSA Measurements In"=w830, "WT1800 Measurements In"=w844, "DSA Averages In"=w846, "WT1800 Averages In"=w849) -> ("DSA Averages Out"=w828:sgl[][], "WT1800 Averages Out"=w847:sgl[][], "Iteration Count Out"=w837:i32)  [unwired: 3 in]
                    n306 = call "DSA Stop AI and AO.vi"("Task ID Cluster"=w852, "error in"=w812, "Buffer Complete"=w809, "WT Errors In"=w811) -> ("AI Task ID Out"=w851:refnum<k21>, "AO Task ID Out"=w850:refnum<k21>[], "errors out"=w825:errorcluster)  [unwired: 13 in]
                    n307 = call "Bundle Measurement Averages.vi"("WT1800 Channel Group"=w829, "WT1800 Measurements"=w847, "DSA Measurements"=w828, "WT1800 Channels per Instrument"=w836, "Number of Functions"=w845) -> ("WT1800 Averages"=w827:T8, "DSA Averages"=w831:T18)  [unwired: 8 in, 1 out]
                    n308 = Merge Errors(w811, w825) -> (w814:errorcluster)
                    n309 = Unbundle By Name(w814) -> ("status"=w848:bool)
                    n310 = Or(x=w848, y="Abort 3") -> (x .or. y?=w821:bool)
                    n311 = Or(x=w809, y=w821) -> (x .or. y?=w835:bool)
                  }
                  n312 = call "Calculate Gains.vi"("DSA Averages"=w771, "WT1800 Averages"=w770, "error in"=w777, "Error or Abort"=w798, "Settings Cluster"=w807) -> ("Gain Array"=w769:T6, "Impedances"=w792:dbl[], "error out"=w803:errorcluster)  [unwired: 6 in, 2 out]
                  n313 = Unbundle By Name(w801) -> ("Frequency Range [Hz].start"=w797:dbl)
                  "Frequency" <- w797
                  n314 = Cluster To Array(cluster=w769) -> (array=w791:dbl[])
                  n315 = call "Bundle EQ and Z Graphs.vi"("Frequency"=w797, "1D Frequency In"=w796, "1D Impedance In"=w792, "2D Impedandce In"=w795, "2D Gain In"=w794, "1D Gain In"=w791) -> ("1D Frequency Out"=w790:dbl[], "2D Impedandce Out"=w789:dbl[][], "2D Gain Out"=w788:dbl[][], "Z Graph"=→"Z Graph":cluster{dbl[], dbl[]}[], "EQ Graph"=→"EQ Graph":cluster{dbl[], dbl[]}[])  [unwired: 1 in]
                }
                frame #1 {
                  w853 = u8 1 ("X Scale.Scale Fit")
                  n316 = property on="EQ Graph" class="XYGraph (strict)"("XScale.ScaleFit"=w853, "YScale.ScaleFit"=w853) -> ()  [unwired: 2 in, 2 out]
                  n317 = property on="Z Graph" class="XYGraph (strict)"("XScale.ScaleFit"=w853, "YScale.ScaleFit"=w853) -> ()  [unwired: 2 in, 2 out]
                }
                frame #2 {
                  n318 = property on="EQ Graph" class="XYGraph (strict)"() -> ("YScale.Maximum"=w867:dbl, "YScale.Minimum"=w857:dbl)  [unwired: 2 in, 2 out]
                  n319 = property on="Z Graph" class="XYGraph (strict)"() -> ("YScale.Maximum"=w864:dbl, "YScale.Minimum"=w856:dbl)  [unwired: 2 in, 2 out]
                  n320 = Subtract(x=w867, y=w857) -> (x-y=w868:dbl)
                  n321 = Subtract(x=w864, y=w856) -> (x-y=w863:dbl)
                  n322 = Divide(x=w868, y=2.0) -> (x/y=w859:dbl)
                  n323 = Divide(x=w863, y=2.0) -> (x/y=w861:dbl)
                  n324 = Add(x=w859, y=w857) -> (x+y=w858:dbl)
                  n325 = Add(x=w861, y=w856) -> (x+y=w860:dbl)
                  n326 = Bundle(1000.0, w858) -> (w866:cluster{dbl, dbl})  [unwired: 1 in]
                  n327 = Bundle(1000.0, w860) -> (w865:cluster{dbl, dbl})  [unwired: 1 in]
                  n328 = property on="EQ Graph" class="XYGraph (strict)"("Cursor.Cursor Position"=w866) -> ()  [unwired: 2 in, 2 out]
                  n329 = property on="Z Graph" class="XYGraph (strict)"("Cursor.Cursor Position"=w865) -> ()  [unwired: 2 in, 2 out]
                }
              }
            }
            frame True {
            }
          }
        }
        n330 = flat-sequence {
          tunnel: w717 -> [w878]
          tunnel: w687 -> [_]
          tunnel: w711 -> [w877]
          frame #0 {
            n331 = property on="Run EQ Check" class="Bool"(error in=w877, "Visible"=w878) -> (error out=w879:errorcluster)  [unwired: 1 in, 1 out]
            n332 = property on="Home" class="Bool"(error in=w879, "Visible"=w878) -> (error out=w876:errorcluster)  [unwired: 1 in, 1 out]
            n333 = Not(x=w878) -> (.not. x?=w880:bool)
            n334 = property on="Abort 3" class="Bool"(error in=w876, "Visible"=w880) -> ()  [unwired: 1 in, 2 out]
          }
        }
        n335 = call "WT1800 Close Instruments.vi"("WT1800 Instruments In"=w688, "Buffer Complete In"=TRUE, "error in"=w687) -> ()  [unwired: 10 in, 3 out]
      }
      frame "Check EQ" {
        w881 = TRUE ("Visible")
        n336 = property on="Home" class="Bool"(error in=w886, "Visible"=w881) -> (error out=w884:errorcluster)  [unwired: 1 in, 1 out]
        n337 = property on="Run EQ Check" class="Bool"(error in=w884, "Visible"=w881) -> (error out=w883:errorcluster)  [unwired: 1 in, 1 out]
        n338 = property on="User Gains" class="Clust (strict)"(error in=w883, "Visible"=w881) -> (error out=w882:errorcluster)  [unwired: 1 in, 1 out]
        n339 = property on="Tab Control" class="TabCtl (strict)"(error in=w882, "Value"=Functions_Tab."EQ Check" ("Tab Control")) -> (error out=w888:errorcluster)  [unwired: 1 in, 1 out]
      }
      frame "Help" {
      }
      frame "Exit" {
        w896 = 0.0 ("Supply Amps")
        w895 = 0.0 ("Supply Volts")
        n340 = local write "Supply Amps"(w896) -> ()
        n341 = local write "Supply Volts"(w895) -> ()
        n342 = Bundle By Name(cluster=w894, "Supply Volts"=w895, "Supply Amps"=w896) -> (w893:T19)
        n343 = call "Read INI.vi"("Settings Cluster In"=w893) -> ("DC Power Supply"=w898:refnum<visa-resource-name>, "Settings Cluster Out"=w897:T21, "Error Out"=w899:errorcluster)  [unwired: 6 in, 10 out]
        n344 = call "Configure DC Power Supply.vi"("DC Power Supply In"=w898, "Error In"=w899, "Settings Cluster"=w897) -> ()  [unwired: 15 in, 2 out]
      }
    }
    n345 = call "Error Module.vi"("error in (no error)"=w22) -> ("error out"=w23:errorcluster)  [unwired: 10 in]
  }
  n346 = while {
    shift-right: [w904] -> w15
    shift-left: w17 -> [w910]
    shift-right: [w909] -> _
    shift-left: w18 -> [w911]
    tunnel: w10 -> [w906]
    tunnel: [w905] -> w9
    stop <- w907 stop-if-true
    n347 = event shown="[0] Timeout" {
      selector: w906 -> [_ _ _ _ _ _ _ _ _ _ _ _ _ _ _]
      dyn-events: [_ _ _ _ _ _ _ _ _ _ _ _ _ _ _] -> w905
      timeout: 500 -> [_ _ _ _ _ _ _ _ _ _ _ _ _ _ _]
      tunnel: w911 -> [w919 w936 w942 w948 w954 w960 w964 w972 w981 w991 w1008 w1014 w1024 w1030 w1033]
      tunnel: w910 -> [w916 w934 w940 w946 w952 w958 w963 w970 w979 w989 w1007 w1013 w1022 w1028 w1032]
      tunnel: [w912 w933 w939 w945 w951 w957 w966 w969 w978 w988 w1010 w1016 w1021 w1027 w1032] -> w903
      tunnel: [w919 w935 w941 w947 w953 w959 w965 w971 w980 w990 w1009 w1015 w1023 w1029 w1033] -> w909
      tunnel: [FALSE ("status") FALSE ("status") FALSE ("status") FALSE ("status") FALSE ("status") FALSE ("status") FALSE ("status") FALSE ("status") FALSE ("status") FALSE ("status") FALSE ("status") FALSE ("status") FALSE ("status") TRUE ("status") w1034] -> w907
      event Timeout {
        n348 = event-data() -> ()  [unwired: 1 in, 1 out]
        n349 = call "Error Module.vi"("Error Module Command"=Error_Module_Command."Report Errors", "error in (no error)"=w916) -> ("error out"=w913:errorcluster)  [unwired: 9 in]
        n350 = call "Error Module.vi"("Error Module Command"=Error_Module_Command."Initialize", "error in (no error)"=w913) -> ("error out"=w912:errorcluster)  [unwired: 9 in]
        n351 = case shown="\"EQ Check\"" "Tab Control" {
          frame "Home", Default {
          }
          frame "Power Test" {
            n352 = property on="Power Graph" class="WFGraph (strict)"() -> ("Cursor.Cursor Plot"=w922:i32)  [unwired: 2 in, 2 out]
            n353 = Increment(x=w922) -> (x+1=→"Power Plot":i32)
            n354 = Boolean To (0,1)(Boolean="P Scale") -> (0, 1=w920:i16)
            n355 = property on="Power Graph" class="WFGraph (strict)"("XScale.ScaleFit"=w920, "YScale.ScaleFit"=w920) -> ()  [unwired: 2 in, 2 out]
          }
          frame "EQ Check" {
            n356 = property on="EQ Graph" class="XYGraph (strict)"() -> ("Cursor.Cursor Plot"=w928:i32)  [unwired: 2 in, 2 out]
            n357 = property on="Z Graph" class="XYGraph (strict)"() -> ("Cursor.Cursor Plot"=w929:i32)  [unwired: 2 in, 2 out]
            n358 = Increment(x=w928) -> (x+1=→"EQ Plot":i32)
            n359 = Increment(x=w929) -> (x+1=→"Z Plot":i32)
            n360 = Boolean To (0,1)(Boolean="EQ Scale") -> (0, 1=w924:i16)
            n361 = Boolean To (0,1)(Boolean="Z Scale") -> (0, 1=w925:i16)
            n362 = property on="EQ Graph" class="XYGraph (strict)"("XScale.ScaleFit"=w924, "YScale.ScaleFit"=w924) -> ()  [unwired: 2 in, 2 out]
            n363 = property on="Z Graph" class="XYGraph (strict)"("XScale.ScaleFit"=w925, "YScale.ScaleFit"=w925) -> ()  [unwired: 2 in, 2 out]
          }
        }
      }
      event "Home": Value Change {
        w937 = T11 {"Command"=enum."Home", "Data"=variant}  # Consumer Control
        n364 = event-data() -> ()  [unwired: 1 in, 1 out]
        n365 = Enqueue Element(queue=w936, element=w937, error in (no error)=w934) -> (queue out=w935:refnum<queue>, error out=w933:errorcluster)  [unwired: 1 in, 1 out]
      }
      event "Supply Set": Value Change {
        w943 = T11 {"Command"=enum."Set DC Supply", "Data"=variant}  # Consumer Control
        n366 = event-data() -> ()  [unwired: 1 in, 1 out]
        n367 = Enqueue Element(queue=w942, element=w943, error in (no error)=w940) -> (queue out=w941:refnum<queue>, error out=w939:errorcluster)  [unwired: 1 in, 1 out]
      }
      event "Range": Value Change {
        w949 = T11 {"Command"=enum."Fixed Range", "Data"=variant}  # Consumer Control
        n368 = event-data() -> ()  [unwired: 1 in, 2 out]
        n369 = Enqueue Element(queue=w948, element=w949, error in (no error)=w946) -> (queue out=w947:refnum<queue>, error out=w945:errorcluster)  [unwired: 1 in, 1 out]
      }
      event "Save Settings": Value Change {
        w955 = T11 {"Command"=enum."Save Settings", "Data"=variant}  # Consumer Control
        n370 = event-data() -> ()  [unwired: 1 in, 1 out]
        n371 = Enqueue Element(queue=w954, element=w955, error in (no error)=w952) -> (queue out=w953:refnum<queue>, error out=w951:errorcluster)  [unwired: 1 in, 1 out]
      }
      event "Load Settings": Value Change {
        w961 = T11 {"Command"=enum."Load Settings", "Data"=variant}  # Consumer Control
        n372 = event-data() -> ()  [unwired: 1 in, 2 out]
        n373 = Enqueue Element(queue=w960, element=w961, error in (no error)=w958) -> (queue out=w959:refnum<queue>, error out=w957:errorcluster)  [unwired: 1 in, 1 out]
      }
      event "Check EQ": Value Change {
        w967 = T11 {"Command"=enum."Check EQ", "Data"=variant}  # Consumer Control
        n374 = event-data() -> ()  [unwired: 1 in, 1 out]
        n375 = Enqueue Element(queue=w964, element=w967, error in (no error)=w963) -> (queue out=w965:refnum<queue>, error out=w966:errorcluster)  [unwired: 1 in, 1 out]
      }
      event "Configure Channels": Value Change {
        w973 = T11 {"Command"=enum."Configure Channels", "Data"=variant}  # Consumer Control
        n376 = event-data() -> ()  [unwired: 1 in, 1 out]
        n377 = Enqueue Element(queue=w972, element=w973, error in (no error)=w970) -> (queue out=w971:refnum<queue>, error out=w969:errorcluster)  [unwired: 1 in, 1 out]
      }
      event "Run Test": Value Change {
        w974 = 0.0 ("Delay Countdown")
        w982 = T11 {"Command"=enum."Run Test", "Data"=variant}  # Consumer Control
        n378 = event-data() -> ()  [unwired: 1 in, 1 out]
        n379 = Enqueue Element(queue=w981, element=w982, error in (no error)=w979) -> (queue out=w980:refnum<queue>, error out=w978:errorcluster)  [unwired: 1 in, 1 out]
        n380 = local write "Delay Countdown"(w974) -> ()
        n381 = local write "V Step"(w974) -> ()
        n382 = local write "Test Countdown"(w974) -> ()
        n383 = local write "Power Graph"(dbl[][] [] ("Graph")) -> ()
        n384 = local write "WT1800"(T8 [{"Vrms"=0.0, "Irms"=0.0, "Power"=0.0, "Vpkpk"=0.0, "Ipkpk"=0.0}, {"Vrms"=0.0, "Irms"=0.0, "Power"=0.0, "Vpkpk"=0.0, "Ipkpk"=0.0}, {"Vrms"=0.0, "Irms"=0.0, "Power"=0.0, "Vpkpk"=0.0, "Ipkpk"=0.0}, {"Vrms"=0.0, "Irms"=0.0, "Power"=0.0, "Vpkpk"=0.0, "Ipkpk"=0.0}, {"Vrms"=0.0, "Irms"=0.0, "Power"=0.0, "Vpkpk"=0.0, "Ipkpk"=0.0}, {"Vrms"=0.0, "Irms"=0.0, "Power"=0.0, "Vpkpk"=0.0, "Ipkpk"=0.0}, {"Vrms"=0.0, "Irms"=0.0, "Power"=0.0, "Vpkpk"=0.0, "Ipkpk"=0.0}, {"Vrms"=0.0, "Irms"=0.0, "Power"=0.0, "Vpkpk"=0.0, "Ipkpk"=0.0}, {"Vrms"=0.0, "Irms"=0.0, "Power"=0.0, "Vpkpk"=0.0, "Ipkpk"=0.0}, {"Vrms"=0.0, "Irms"=0.0, "Power"=0.0, "Vpkpk"=0.0, "Ipkpk"=0.0}, {"Vrms"=0.0, "Irms"=0.0, "Power"=0.0, "Vpkpk"=0.0, "Ipkpk"=0.0}, {"Vrms"=0.0, "Irms"=0.0, "Power"=0.0, "Vpkpk"=0.0, "Ipkpk"=0.0}, {"Vrms"=0.0, "Irms"=0.0, "Power"=0.0, "Vpkpk"=0.0, "Ipkpk"=0.0}, {"Vrms"=0.0, "Irms"=0.0, "Power"=0.0, "Vpkpk"=0.0, "Ipkpk"=0.0}, {"Vrms"=0.0, "Irms"=0.0, "Power"=0.0, "Vpkpk"=0.0, "Ipkpk"=0.0}, {"Vrms"=0.0, "Irms"=0.0, "Power"=0.0, "Vpkpk"=0.0, "Ipkpk"=0.0}, {"Vrms"=0.0, "Irms"=0.0, "Power"=0.0, "Vpkpk"=0.0, "Ipkpk"=0.0}, {"Vrms"=0.0, "Irms"=0.0, "Power"=0.0, "Vpkpk"=0.0, "Ipkpk"=0.0}] ("WT1800")) -> ()
      }
      event "Run Configuration": Value Change {
        n385 = event-data() -> ()  [unwired: 1 in, 1 out]
        n386 = local read "Channel List"() -> (w985:T3)
        n387 = Cluster To Array(cluster=w985) -> (array=w986:T5[])
        n388 = for {
          tunnel: [w993] -> w984 mode=indexing
          tunnel: w986 -> [w995] mode=indexing
          w992 = enum16{"---", "1", "1 AVG", "2", "2 AVG"}."---"  # Input
          n389 = Unbundle By Name(w995) -> ("Input"=w994:T26)
          n390 = Equal?(x=w992, y=w994) -> (x = y?=w993:bool)
        }
        n391 = And Array Elements(Boolean array=w984) -> (logical AND=w983:bool)
        n392 = case shown="False" w983 {
          tunnel: w991 -> [w1001 w1005]
          tunnel: [w1000 w1005] -> w990
          tunnel: w989 -> [w999 w1004]
          tunnel: [w998 w1004] -> w988
          frame False {
            w996 = T1 {"Gain 1"=0.0, "Gain 2"=0.0, "Gain 3"=0.0, "Gain 4"=0.0, "Gain 5"=0.0, "Gain 6"=0.0} ("User Gains")
            w1002 = T11 {"Command"=enum."Run Configuration", "Data"=variant}  # Consumer Control
            n393 = Enqueue Element(queue=w1001, element=w1002, error in (no error)=w999) -> (queue out=w1000:refnum<queue>, error out=w998:errorcluster)  [unwired: 1 in, 1 out]
            n394 = local write "User Gains"(w996) -> ()
            n395 = local write "Gain Averages"(w996) -> ()
            n396 = local write "Gain Array"(T6 {"Gain 1"=0.0, "Gain 2"=0.0, "Gain 3"=0.0, "Gain 4"=0.0, "Gain 5"=0.0, "Gain 6"=0.0, "Gain 7"=0.0, "Gain 8"=0.0, "Gain 9"=0.0, "Gain 10"=0.0, "Gain 11"=0.0, "Gain 12"=0.0, "Gain 13"=0.0, "Gain 14"=0.0, "Gain 15"=0.0, "Gain 16"=0.0, "Gain 17"=0.0} ("Gain Array")) -> ()
          }
          frame True {
            n397 = One Button Dialog(message="Please Select at least 1 input channel.") -> ()  [unwired: 1 in, 1 out]
          }
        }
      }
      event "Power Test": Value Change {
        w1011 = T11 {"Command"=enum."Power Test", "Data"=variant}  # Consumer Control
        n398 = event-data() -> ()  [unwired: 1 in, 1 out]
        n399 = Enqueue Element(queue=w1008, element=w1011, error in (no error)=w1007) -> (queue out=w1009:refnum<queue>, error out=w1010:errorcluster)  [unwired: 1 in, 1 out]
      }
      event "Power Test M": Value Change {
        w1017 = T11 {"Command"=enum."Power Test M", "Data"=variant}  # Consumer Control
        n400 = event-data() -> ()  [unwired: 1 in, 1 out]
        n401 = Enqueue Element(queue=w1014, element=w1017, error in (no error)=w1013) -> (queue out=w1015:refnum<queue>, error out=w1016:errorcluster)  [unwired: 1 in, 1 out]
      }
      event "Run EQ Check": Value Change {
        w1019 = cluster{dbl[], "Gain Array":dbl[]}[] [] ("EQ Graph")
        w1025 = T11 {"Command"=enum."Run EQ", "Data"=variant}  # Consumer Control
        n402 = event-data() -> ()  [unwired: 1 in, 1 out]
        n403 = Enqueue Element(queue=w1024, element=w1025, error in (no error)=w1022) -> (queue out=w1023:refnum<queue>, error out=w1021:errorcluster)  [unwired: 1 in, 1 out]
        n404 = local write "EQ Graph"(w1019) -> ()
        n405 = local write "Z Graph"(w1019) -> ()
        n406 = local write "Frequency"(0.0 ("Frequency [Hz]")) -> ()
      }
      event "Exit": Value Change {
        w1031 = T11 {"Command"=enum."Exit", "Data"=variant}  # Consumer Control
        n407 = event-data() -> ()  [unwired: 1 in, 1 out]
        n408 = Enqueue Element(queue=w1030, element=w1031, error in (no error)=w1028) -> (queue out=w1029:refnum<queue>, error out=w1027:errorcluster)  [unwired: 1 in, 1 out]
      }
      event User Event {
        n409 = event-data() -> ("status"=w1034:bool)  [unwired: 1 in]
      }
    }
    n410 = call "Error Module.vi"("error in (no error)"=w903) -> ("error out"=w904:errorcluster)  [unwired: 10 in]
  }
  n411 = Release Queue(queue=w14, error in (no error)=w13) -> (error out=w12:errorcluster)  [unwired: 1 in, 2 out]
  n412 = Merge Errors(w15, w12) -> (w5:errorcluster)
  n413 = Unregister For Events(event registration refnum=w9, error in=w5) -> (error out=w6:errorcluster)
  n414 = Destroy User Event(user event=w7, error in=w6) -> (error out=w4:errorcluster)
  n415 = flat-sequence {
    tunnel: w1 -> [_]
    frame #0 {
      n416 = Quit LabVIEW(quit? (T)=TRUE) -> ()
    }
  }
  n417 = call "Error Module.vi"("Error Module Command"=Error_Module_Command."Report Errors", "error in (no error)"=w4) -> ("error out"=w1:errorcluster)  [unwired: 9 in]
